vi "ClosedLoop+OpenWindLightOdor_v3.vi"() -> ()   [LabVIEW 2014]
uses:
  <vilib>/vision/Measure.llb/Straight Edge Options.ctl
  <vilib>/vision/Measure.llb/Straight Edge Process.ctl
  <vilib>/Platform/TimedLoop/XDataNode/timing_clust.ctl
  <vilib>/Platform/TimedLoop/XDataNode/nitl_modes.ctl
  <vilib>/Platform/TimedLoop/XDataNode/wakeup.ctl
  <vilib>/vision/Measure.llb/Edge Options.ctl
  <vilib>/vision/Measure.llb/Edge Polarity.ctl
  <vilib>/gmath/statdist.llb/Random Permutation.vi
  <vilib>/DAQmx/create/channels.llb/DAQmx Create Channel (DO-Digital Output).vi
  <vilib>/DAQmx/write.llb/DAQmx Write (Digital Bool 1Line 1Point).vi
  <vilib>/gmath/statdist.llb/Uniform (Discrete) Random.vi
  <vilib>/DAQmx/create/channels.llb/DAQmx Create Channel (AO-Voltage-Basic).vi
  <vilib>/Platform/TimedLoop/TimeConversion.llb/rt-rel-time-to-milliseconds.vi
  <vilib>/DAQmx/write.llb/DAQmx Write (Analog DBL 1Chan 1Samp).vi
  <vilib>/DAQmx/create/channels.llb/DAQmx Create Channel (DI-Digital Input).vi
  <vilib>/DAQmx/read.llb/DAQmx Read (Digital Bool 1Line 1Point).vi
  <vilib>/platform/TimedLoop/XDataNode/XDataNode.xnode
  <vilib>/vision/driver/NI_Vision_Acquisition_Software.lvlib
  <vilib>/Platform/TimedLoop/XDataNode/XDNodeRunTimeDep.lvlib
  <vilib>/vision/NI_Vision_Development_Module.lvlib
  <vilib>/gmath/NI_Gmath.lvlib
panel:
  out "Wind Intensity (V)":dbl=5.0
  out "Wind Trial":bool
  out "head ind":i32
  out "Slide 5":dbl(slide) scale=0.0..1.0
  out "Slide 4":dbl(slide) scale=0.0..1.0
  out "Slide 3":dbl(slide) scale=0.0..1.0
  out "Slide 2":dbl(slide) scale=0.0..1.0
  out "Light Trial":bool
  in  "Vary Stimulus Intensity":bool
  out "Cond. 4":i32
  out "Cond. 3":i32
  out "Cond. 2":i32
  out "Cond. 1":i32
  out "Light Intensity (V)":dbl=5.0
  in  "Rand light":bool
  in  "Use light?":bool
  in  "Reversed Tether?":bool=TRUE
  in  "R options":T1={"Number of Lines"=1, "Type"=enum."Best Edge Projection", "Min. Score"=10.0, "Max. Score"=1000.0, "Orientation"=-135.0, "Angle Range"=45.0, "Angle Tolerance"=1.0, "Step Size"=3, "Min. SNR (db)"=0.0, "Min. Points (%)"=25.0, "Hough Iterations"=3} {"Min. Points (%)" min=0.0 max=100.0; "Min. SNR (db)" min=0.0; "Max. Score" min=0.0 max=1024.0; "Min. Score" min=0.0 max=1024.0 step=1.0}
  in  "L options":T1={"Number of Lines"=1, "Type"=enum."Best Edge Projection", "Min. Score"=10.0, "Max. Score"=1000.0, "Orientation"=135.0, "Angle Range"=45.0, "Angle Tolerance"=1.0, "Step Size"=3, "Min. SNR (db)"=0.0, "Min. Points (%)"=25.0, "Hough Iterations"=3} {"Min. Points (%)" min=0.0 max=100.0; "Min. SNR (db)" min=0.0; "Max. Score" min=0.0 max=1024.0; "Min. Score" min=0.0 max=1024.0 step=1.0}
  in  "Rand wind":bool
  in  "Use wind?":bool=TRUE
  in  "Use odor?":bool
  in  "Pre-Spec. H(0)":bool=TRUE
  out "X (steps/sample)":dbl(graph)
  out "Slide":dbl(slide) scale=0.0..1.0
  out "Motor Error":bool
  in  "Max steps/sample":dbl=6.0
  in  "Step Rate (Hz)":dbl=500.0
  out "Heading (deg)":dbl(graph)
  out "H":dbl format="%.4f"
  out "X (steps/sample)":dbl
  in  "Geneotype":string="w1118"
  out "Odor On":bool
  in  "Starvation Time (hrs)":string="1"
  in  "Age (DSE)":string="4"
  out "Trial End":bool
  in  "Trial Duration (s)":dbl=60.0
  out "Odor Duration (s)":dbl=10.0
  in  "Odor Onset Time (s)":dbl=90.0
  out "Trial":i32 format="%#.3f"
  in  "Number of Trials":i32=20
  in  "Experiment name":string="E1"
  in  "Fly ID":string
  in  "L-R WBA Offset (deg)":dbl format="%#_13g"
  in  "deltaWBA Scale Factor (k, unitless)":dbl=0.04 format="%.4f"
  out "L-R WBA":dbl
  out "deltaWBA":dbl format="%.4f"
  out "Scaled deltaWBA (deg)":dbl(graph)
  out "R WBA":dbl
  out "L WBA":dbl
  out "Image":T3(plugin-control)
  in  "Image Threshold":cluster{"Lower value":sgl, "Upper value":sgl}={"Lower value"=110.0, "Upper value"=255.0} {"Upper value" format="%.2f"; "Lower value" format="%.2f"}
  in  "Data Rate (Hz)":dbl=50.0
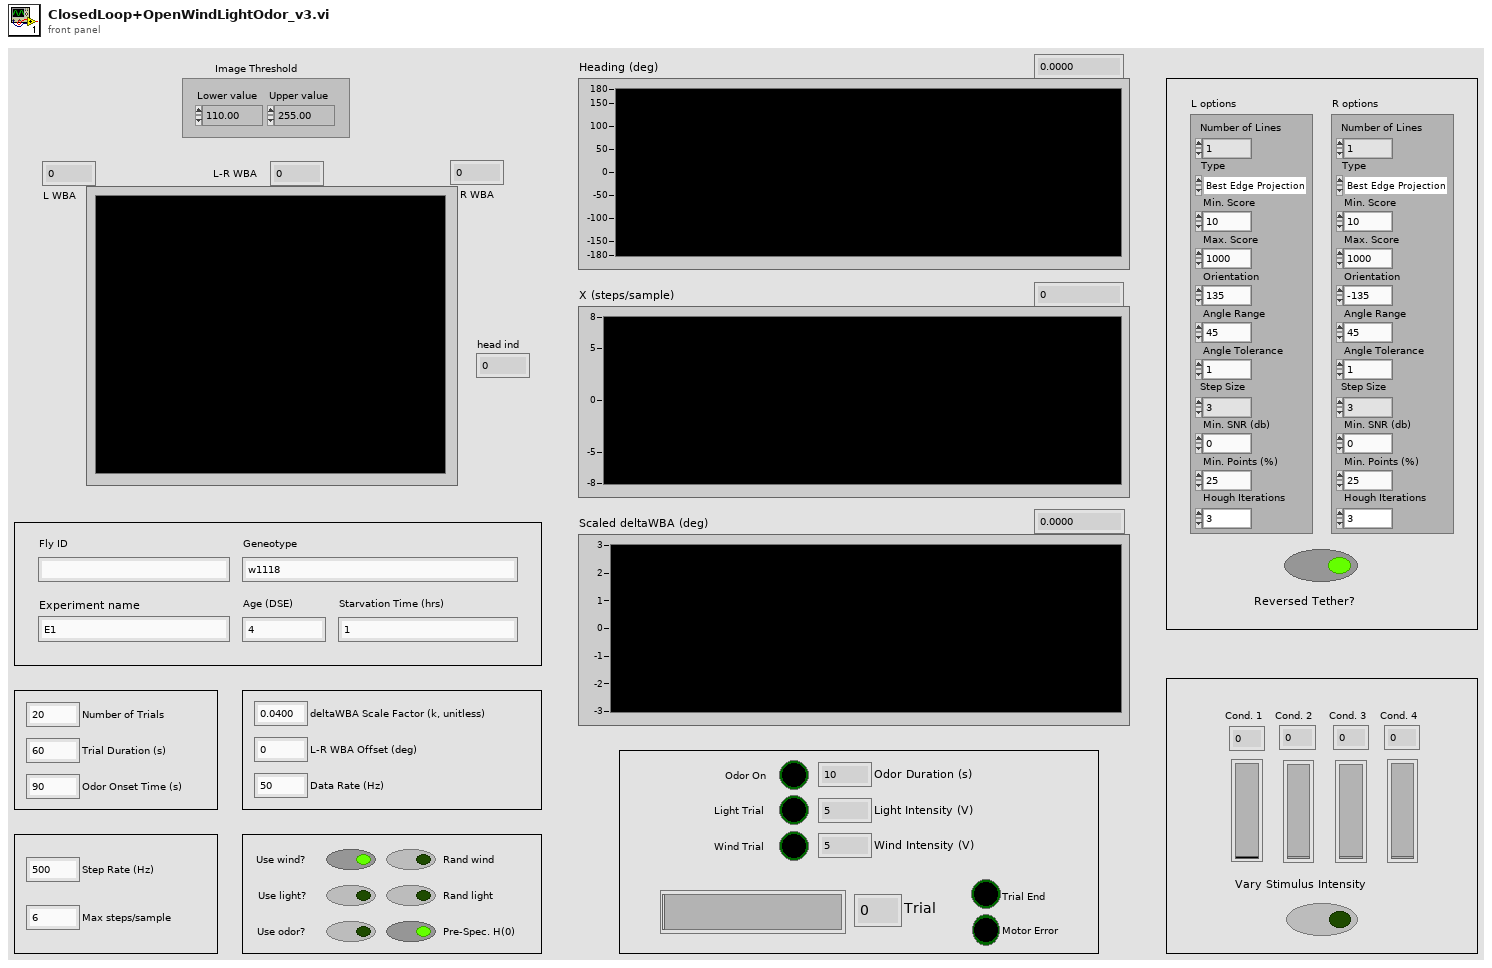
[diagram p1: front panel]
types:
  T1 = typedef "Straight Edge Options.ctl" = cluster{"Number of Lines":i32, "Type":T2, "Min. Score":dbl, "Max. Score":dbl, "Orientation":dbl, "Angle Range":dbl, "Angle Tolerance":dbl, "Step Size":u32, "Min. SNR (db)":dbl, "Min. Points (%)":dbl, "Hough Iterations":i32}
  T2 = typedef "Straight Edge Process.ctl" = enum32{"First Edge Rake", "Best Edge Rake", "Hough Edge Rake", "First Edge Projection", "Best Edge Projection"}
  T3 = typedef "IMAQ Image.ctl" = refnum<image>
  T4 = enum16{"open", "replace", "create", "open or create", "replace or create", "replace or create with confirmation"}
  T5 = typedef "IMAQdx.ctl" = refnum<k21>
  T6 = typedef "IMAQ Rectangle" = cluster{"Left":i32, "Top":i32, "Right":i32, "Bottom":i32, "Rotation":dbl}
  T7 = typedef "ROI Descriptor" = cluster{"Global Rectangle":i32[], "Contours":cluster{"ID":enum32{"External", "Internal"}, "Type":u32, "Coordinates":i32[]}[]}
  T8 = typedef "XDNodeRunTimeDep.lvlib/timing_clust.ctl" = cluster{"Expected End [f-1]":u64, "Actual End [f-1]":u64, "Finished Late? [f-1]":bool, "Expected End [i-1]":u64, "Actual End [i-1]":u64, "Finished Late? [i-1]":bool, "Expected Start [i]":u64, "Actual Start [i]":u64, "Expected Start [f]":u64, "Actual Start [f]":u64, "Source Name":string, "Structure Name":string, "Period":i64, "Deadline":i64, "Offset":i64, "Start":i64, "Priority":i32, "Timeout":i32, "Mode":T9, "Wakeup Reason":T10, "Error":errorcluster, "Source Type":string, "Secondary Source Type":string, "Global End Time":u64, "Global Start Time":u64, "Frame Duration":u64, "Iteration Duration":u64, "Assigned CPU":i32, "I/O Scan Engine Mode":u32}
  T9 = typedef "XDNodeRunTimeDep.lvlib/nitl_modes.ctl" = enum32{"No Change", "Process missed periods, maintain original phase", "Discard missed periods, maintain original phase", "Process missed periods, ignore original phase", "Discard missed periods, ignore original phase"}
  T10 = typedef "XDNodeRunTimeDep.lvlib/wakeup.ctl" = enum32{"Normal", "Aborted", "Asynchronous wakeup", "Timing source error", "Timed loop error", "Timeout"}
  T11 = typedef "Edge Options.ctl" = cluster{"Edge Polarity":T12, "Kernel Size":u32, "Width":u32, "Minimum Edge Strength":sgl, "Interpolation Type":enum32{"Zero Order", "Bilinear", "Quadratic", "Cubic", "Bilinear Fixed"}, "Data Processing Method":enum32{"Average", "Median"}}
  T12 = typedef "Edge Polarity.ctl" = u32
  T13 = cluster{"Search Direction":u32, "Edge Options":T11, "Show Search Area":bool, "Show Search Lines":bool, "Show Edges Found":bool, "Show Result":bool, "Search Area Color":u32, "Search Lines Color":u32, "Edge Locations Color":u32, "Result Color":u32, "Overlay Group Name":string}
  T14 = cluster{"Point1 (Pixels)":cluster{"X":sgl, "Y":sgl}, "Point2 (Pixels)":cluster{"X":sgl, "Y":sgl}, "Point1 (Real-World)":cluster{"X":sgl, "Y":sgl}, "Point2 (Real-World)":cluster{"X":sgl, "Y":sgl}, "Angle (Pixel)":dbl, "Angle (Real-World)":dbl, "Score":dbl, "Straightness":dbl, "Average SNR (db)":dbl, "Calibration Valid":bool}[]
  T15 = cluster{"Straight Edges[0]":cluster{"Point1 (Pixels)":cluster{"X":sgl, "Y":sgl}, "Point2 (Pixels)":cluster{"X":sgl, "Y":sgl}, "Point1 (Real-World)":cluster{"X":sgl, "Y":sgl}, "Point2 (Real-World)":cluster{"X":sgl, "Y":sgl}, "Angle (Pixel)":dbl, "Angle (Real-World)":dbl, "Score":dbl, "Straightness":dbl, "Average SNR (db)":dbl, "Calibration Valid":bool}, "Straight Edges[1]":cluster{"Point1 (Pixels)":cluster{"X":sgl, "Y":sgl}, "Point2 (Pixels)":cluster{"X":sgl, "Y":sgl}, "Point1 (Real-World)":cluster{"X":sgl, "Y":sgl}, "Point2 (Real-World)":cluster{"X":sgl, "Y":sgl}, "Angle (Pixel)":dbl, "Angle (Real-World)":dbl, "Score":dbl, "Straightness":dbl, "Average SNR (db)":dbl, "Calibration Valid":bool}, "Straight Edges[2]":cluster{"Point1 (Pixels)":cluster{"X":sgl, "Y":sgl}, "Point2 (Pixels)":cluster{"X":sgl, "Y":sgl}, "Point1 (Real-World)":cluster{"X":sgl, "Y":sgl}, "Point2 (Real-World)":cluster{"X":sgl, "Y":sgl}, "Angle (Pixel)":dbl, "Angle (Real-World)":dbl, "Score":dbl, "Straightness":dbl, "Average SNR (db)":dbl, "Calibration Valid":bool}, "Straight Edges[3]":cluster{"Point1 (Pixels)":cluster{"X":sgl, "Y":sgl}, "Point2 (Pixels)":cluster{"X":sgl, "Y":sgl}, "Point1 (Real-World)":cluster{"X":sgl, "Y":sgl}, "Point2 (Real-World)":cluster{"X":sgl, "Y":sgl}, "Angle (Pixel)":dbl, "Angle (Real-World)":dbl, "Score":dbl, "Straightness":dbl, "Average SNR (db)":dbl, "Calibration Valid":bool}, "Straight Edges[4]":cluster{"Point1 (Pixels)":cluster{"X":sgl, "Y":sgl}, "Point2 (Pixels)":cluster{"X":sgl, "Y":sgl}, "Point1 (Real-World)":cluster{"X":sgl, "Y":sgl}, "Point2 (Real-World)":cluster{"X":sgl, "Y":sgl}, "Angle (Pixel)":dbl, "Angle (Real-World)":dbl, "Score":dbl, "Straightness":dbl, "Average SNR (db)":dbl, "Calibration Valid":bool}, "Straight Edges[5]":cluster{"Point1 (Pixels)":cluster{"X":sgl, "Y":sgl}, "Point2 (Pixels)":cluster{"X":sgl, "Y":sgl}, "Point1 (Real-World)":cluster{"X":sgl, "Y":sgl}, "Point2 (Real-World)":cluster{"X":sgl, "Y":sgl}, "Angle (Pixel)":dbl, "Angle (Real-World)":dbl, "Score":dbl, "Straightness":dbl, "Average SNR (db)":dbl, "Calibration Valid":bool}, "Straight Edges[6]":cluster{"Point1 (Pixels)":cluster{"X":sgl, "Y":sgl}, "Point2 (Pixels)":cluster{"X":sgl, "Y":sgl}, "Point1 (Real-World)":cluster{"X":sgl, "Y":sgl}, "Point2 (Real-World)":cluster{"X":sgl, "Y":sgl}, "Angle (Pixel)":dbl, "Angle (Real-World)":dbl, "Score":dbl, "Straightness":dbl, "Average SNR (db)":dbl, "Calibration Valid":bool}, "Straight Edges[7]":cluster{"Point1 (Pixels)":cluster{"X":sgl, "Y":sgl}, "Point2 (Pixels)":cluster{"X":sgl, "Y":sgl}, "Point1 (Real-World)":cluster{"X":sgl, "Y":sgl}, "Point2 (Real-World)":cluster{"X":sgl, "Y":sgl}, "Angle (Pixel)":dbl, "Angle (Real-World)":dbl, "Score":dbl, "Straightness":dbl, "Average SNR (db)":dbl, "Calibration Valid":bool}, "Straight Edges[8]":cluster{"Point1 (Pixels)":cluster{"X":sgl, "Y":sgl}, "Point2 (Pixels)":cluster{"X":sgl, "Y":sgl}, "Point1 (Real-World)":cluster{"X":sgl, "Y":sgl}, "Point2 (Real-World)":cluster{"X":sgl, "Y":sgl}, "Angle (Pixel)":dbl, "Angle (Real-World)":dbl, "Score":dbl, "Straightness":dbl, "Average SNR (db)":dbl, "Calibration Valid":bool}}
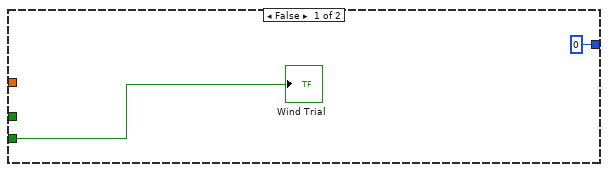
[diagram p2: hidden frame]
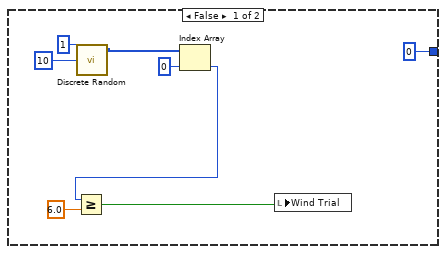
[diagram p3: hidden frame]
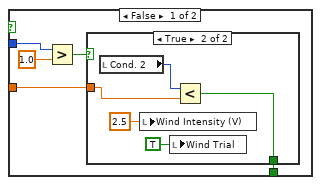
[diagram p4: hidden frame]
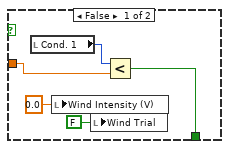
[diagram p5: hidden frame]
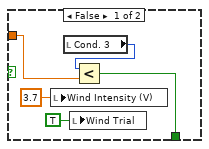
[diagram p6: hidden frame]
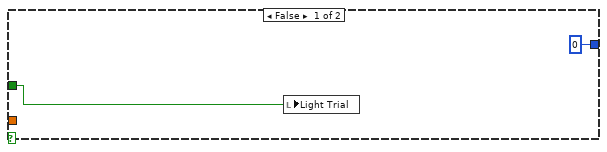
[diagram p7: hidden frame]
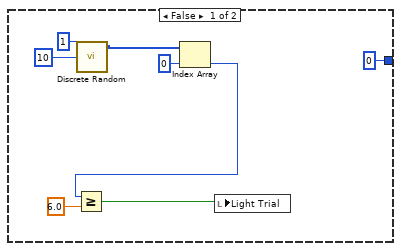
[diagram p8: hidden frame]
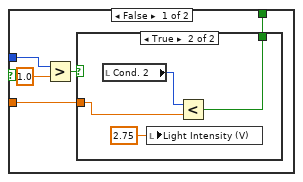
[diagram p9: hidden frame]
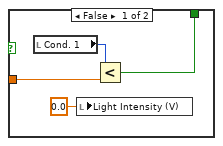
[diagram p10: hidden frame]
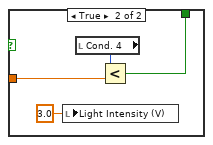
[diagram p11: hidden frame]
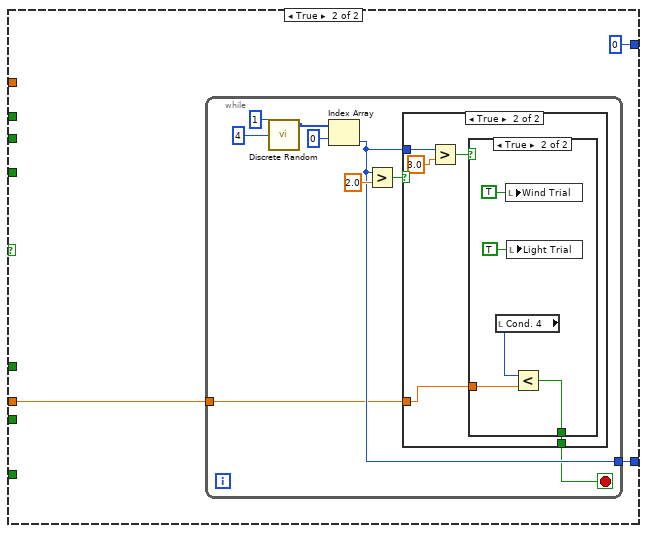
[diagram p12: hidden frame]
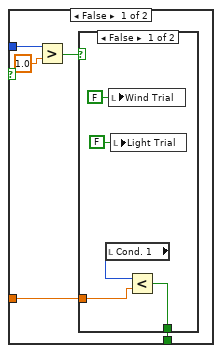
[diagram p13: hidden frame]
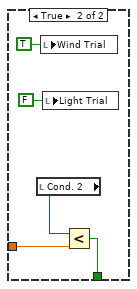
[diagram p14: hidden frame]
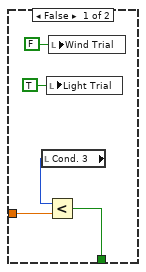
[diagram p15: hidden frame]
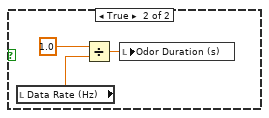
[diagram p17: hidden frame]
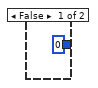
[diagram p19: hidden frame]
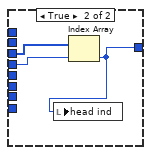
[diagram p20: hidden frame]
diagram:
  w123 = "."
  w125 = "."
  n1 = Boolean To (0,1)(Boolean="Use odor?") -> (0, 1=w86:i16)
  n2 = Boolean To (0,1)(Boolean="Use wind?") -> (0, 1=w75:i16)
  n3 = Boolean To (0,1)(Boolean="Vary Stimulus Intensity") -> (0, 1=w33:i16)
  n4 = Boolean To (0,1)(Boolean="Rand wind") -> (0, 1=w71:i16)
  n5 = Boolean To (0,1)(Boolean="Use light?") -> (0, 1=w50:i16)
  n6 = Boolean To (0,1)(Boolean="Rand light") -> (0, 1=w46:i16)
  n7 = local read "deltaWBA Scale Factor (k, unitless)"() -> (w100:dbl)
  n8 = local read "Data Rate (Hz)"() -> (w101:dbl)
  n9 = local read "Odor Onset Time (s)"() -> (w106:dbl)
  n10 = local read "Trial Duration (s)"() -> (w109:dbl)
  n11 = local read "Number of Trials"() -> (w111:i32)
  n12 = To Double Precision Float(number=w86) -> (double precision float=w85:dbl)
  n13 = To Double Precision Float(number=w75) -> (double precision float=w74:dbl)
  n14 = To Double Precision Float(number=w33) -> (double precision float=w31:dbl)
  n15 = To Double Precision Float(number=w71) -> (double precision float=w69:dbl)
  n16 = local read "Max steps/sample"() -> (w98:dbl)
  n17 = To Double Precision Float(number=w50) -> (double precision float=w48:dbl)
  n18 = To Double Precision Float(number=w46) -> (double precision float=w44:dbl)
  n19 = local read "Step Rate (Hz)"() -> (w99:dbl)
  n20 = local read "Reversed Tether?"() -> (w54:bool)
  n21 = Boolean To (0,1)(Boolean=w54) -> (0, 1=w55:i16)
  n22 = To Double Precision Float(number=w55) -> (double precision float=w53:dbl)
  n23 = Number To Fractional String(number=w111, precision (6)=i16 0) -> (F-format string=w92:string)  [unwired: 2 in]
  n24 = Number To Fractional String(number=w109, precision (6)=i16 0) -> (F-format string=w91:string)  [unwired: 2 in]
  n25 = Number To Fractional String(number=w106, precision (6)=i16 0) -> (F-format string=w90:string)  [unwired: 2 in]
  n26 = Number To Fractional String(number=w85, precision (6)=i16 0) -> (F-format string=w89:string)  [unwired: 2 in]
  n27 = Number To Fractional String(number=w74, precision (6)=i16 0) -> (F-format string=w73:string)  [unwired: 2 in]
  n28 = Number To Fractional String(number=w101, precision (6)=i16 0) -> (F-format string=w67:string)  [unwired: 2 in]
  n29 = Number To Fractional String(number=w99, precision (6)=i16 0) -> (F-format string=w66:string)  [unwired: 2 in]
  n30 = Number To Fractional String(number=w98, precision (6)=i16 0) -> (F-format string=w65:string)  [unwired: 2 in]
  n31 = Number To Fractional String(number=w100, precision (6)=i16 3) -> (F-format string=w64:string)  [unwired: 2 in]
  n32 = Number To Fractional String(number=w31, precision (6)=i16 0) -> (F-format string=w30:string)  [unwired: 2 in]
  n33 = Number To Fractional String(number=w69, precision (6)=i16 0) -> (F-format string=w68:string)  [unwired: 2 in]
  n34 = Number To Fractional String(number=w53, precision (6)=i16 0) -> (F-format string=w52:string)  [unwired: 2 in]
  n35 = Number To Fractional String(number=w48, precision (6)=i16 0) -> (F-format string=w36:string)  [unwired: 2 in]
  n36 = Number To Fractional String(number=w44, precision (6)=i16 0) -> (F-format string=w35:string)  [unwired: 2 in]
  n37 = Get Date/Time In Seconds() -> (seconds since 1Jan1904=w131:timestamp)
  n38 = Get Date/Time In Seconds() -> (seconds since 1Jan1904=w127:timestamp)
  n39 = Get Date/Time In Seconds() -> (seconds since 1Jan1904=w129:timestamp)
  n40 = call <vilib>:"Space Constant.vi"() -> ("String"=w133:string)
  n41 = Format Date/Time String(time format string (%c)="%d", seconds (now)=w131) -> (date/time string=w122:string)  [unwired: 1 in]
  n42 = Format Date/Time String(time format string (%c)="%m", seconds (now)=w129) -> (date/time string=w124:string)  [unwired: 1 in]
  n43 = Format Date/Time String(time format string (%c)="%Y", seconds (now)=w127) -> (date/time string=w126:string)  [unwired: 1 in]
  n44 = Concatenate Strings(w126, w125, w124, w123, w122) -> (w97:string)
  n45 = Concatenate Strings(w126, w125, w124, w123, w122, w133, "fly_", "Fly ID", "\\") -> (w137:string)
  n46 = String To Path(string=w137) -> (path=w136:path)
  n47 = Build Path(base path=path "E:/TAC DATA ARCHIVE/NewRig/labview/ClosedLoop+OpenWindLightOdor", name or relative path=w136) -> (appended path=w141:path)
  n48 = call <vilib>:"IMAQdx Open Camera.vi"("Session In"=refnum<k21> "cam8" ("Camera Name")) -> ("Session Out"=w163:T5)  [unwired: 2 in, 8 out]
  n49 = call <vilib>:"Check if File or Folder Exists.vi"("path"=w141) -> ("file or folder exists?"=w139:bool, "dup path"=w140:path)  [unwired: 8 in, 1 out]
  n50 = call <vilib>:"IMAQdx Configure Grab.vi"("Session In"=w163) -> ("Session Out"=w161:T5)  [unwired: 1 in, 9 out]
  n51 = case shown="False" w139 {
    tunnel: w140 -> [w165 w166]
    tunnel: [w164 w166] -> w145
    frame False {
      n52 = Create Folder(path (use dialog)=w165) -> (created path=w164:path)  [unwired: 2 in, 2 out]
    }
    frame True {
    }
  }
  n53 = call "IMAQ Create"("Image Name"="ROIR") -> ("New Image"=w160:T3)  [unwired: 3 in, 2 out]
  n54 = Concatenate Strings("Experiment name", "\\") -> (w113:string)
  n55 = call <vilib>:"IMAQdx Grab.vi"("Image In"=w160, "Session In"=w161) -> ("Image Out"=w159:T3, "Session Out"=w150:T5)  [unwired: 2 in, 6 out]
  n56 = String To Path(string=w113) -> (path=w142:path)
  n57 = call "IMAQ Select Rectangle"("Prompt"="Select RIGHT ROI for wing angle detection", "Image In"=w159) -> ("Rectangle"=w151:T6)  [unwired: 6 in, 3 out]
  n58 = Build Path(base path=w145, name or relative path=w142) -> (appended path=w146:path)
  n59 = call "IMAQ Convert Rectangle to ROI"("Rectangle"=w151) -> ("ROI Descriptor"=w149:T7)  [unwired: 8 in, 1 out]
  n60 = call <vilib>:"Check if File or Folder Exists.vi"("path"=w146) -> ("file or folder exists?"=w143:bool, "dup path"=w144:path)  [unwired: 8 in, 1 out]
  n61 = call "IMAQ Create"("Image Name"="ROIL") -> ("New Image"=w155:T3)  [unwired: 3 in, 2 out]
  n62 = case shown="False" w143 {
    tunnel: w144 -> [w168 w169]
    tunnel: [w167 w169] -> w1
    frame False {
      n63 = Create Folder(path (use dialog)=w168) -> (created path=w167:path)  [unwired: 2 in, 2 out]
    }
    frame True {
    }
  }
  n64 = call <vilib>:"IMAQdx Grab.vi"("Image In"=w155, "Session In"=w150) -> ("Image Out"=w154:T3, "Session Out"=w148:T5)  [unwired: 2 in, 6 out]
  n65 = String To Path(string="experiment_information") -> (path=w121:path)
  n66 = call "IMAQ Select Rectangle"("Prompt"="Select LEFT ROI for wing angle detection", "Image In"=w154) -> ("Rectangle"=w156:T6)  [unwired: 6 in, 3 out]
  n67 = Build Path(base path=w1, name or relative path=w121) -> (appended path=w118:path)
  n68 = String To Path(string="odor_durations") -> (path=w84:path)
  n69 = String To Path(string="light_intensities") -> (path=w43:path)
  n70 = String To Path(string="wind_boolean") -> (path=w63:path)
  n71 = String To Path(string="wind_intensities") -> (path=w10:path)
  n72 = call "IMAQ Convert Rectangle to ROI"("Rectangle"=w156) -> ("ROI Descriptor"=w147:T7)  [unwired: 8 in, 1 out]
  n73 = Build Path(base path=w1, name or relative path=w84) -> (appended path=w81:path)
  n74 = Build Path(base path=w1, name or relative path=w43) -> (appended path=w40:path)
  n75 = Build Path(base path=w1, name or relative path=w63) -> (appended path=w60:path)
  n76 = Build Path(base path=w1, name or relative path=w10) -> (appended path=w7:path)
  n77 = Open/Create/Replace File(file path (use dialog)=w118, operation (0:open)=T4."create", access (0:read/write)=enum16{"read/write", "read-only", "write-only"}."write-only") -> (refnum out=w116:refnum<file>)  [unwired: 3 in, 2 out]
  n78 = Open/Create/Replace File(file path (use dialog)=w81, operation (0:open)=T4."create", access (0:read/write)=enum16{"read/write", "read-only", "write-only"}."write-only") -> (refnum out=w79:refnum<file>)  [unwired: 3 in, 2 out]
  n79 = Open/Create/Replace File(file path (use dialog)=w40, operation (0:open)=T4."create", access (0:read/write)=enum16{"read/write", "read-only", "write-only"}."write-only") -> (refnum out=w38:refnum<file>)  [unwired: 3 in, 2 out]
  n80 = Open/Create/Replace File(file path (use dialog)=w60, operation (0:open)=T4."create", access (0:read/write)=enum16{"read/write", "read-only", "write-only"}."write-only") -> (refnum out=w58:refnum<file>)  [unwired: 3 in, 2 out]
  n81 = Open/Create/Replace File(file path (use dialog)=w7, operation (0:open)=T4."create", access (0:read/write)=enum16{"read/write", "read-only", "write-only"}."write-only") -> (refnum out=w5:refnum<file>)  [unwired: 3 in, 2 out]
  n82 = Build Array(w97, "Fly ID", "Experiment name", "Age (DSE)", "Starvation Time (hrs)", w92, w91, w90, w89, w73, w68, w67, w66, w65, w64, w52, w36, w35, w30, "Geneotype") -> (w88:string[])
  n83 = Write to Text File(file (use dialog)=w116, text=w88) -> (refnum out=w115:refnum<file>)  [unwired: 2 in, 2 out]
  n84 = Close File(refnum=w115) -> ()  [unwired: 1 in, 2 out]
  n85 = flat-sequence {
    tunnel: w1 -> [w175]
    tunnel: w147 -> [w176]
    tunnel: w148 -> [w177]
    tunnel: w149 -> [w178]
    tunnel: [w178] -> w28
    tunnel: [w177] -> w26
    tunnel: [w176] -> w24
    tunnel: [w175] -> w22
    tunnel: [w173] -> w20
    tunnel: w79 -> [w173]
    tunnel: [w172] -> w18
    tunnel: w58 -> [w172]
    tunnel: w38 -> [w171]
    tunnel: [w171] -> w16
    tunnel: w5 -> [w170]
    tunnel: [w170] -> w4
    tunnel: w28 -> [w193]
    tunnel: [w193] -> w27
    tunnel: w26 -> [w192]
    tunnel: [w192] -> w25
    tunnel: w24 -> [w191]
    tunnel: [w191] -> w23
    tunnel: w22 -> [w190]
    tunnel: [w190] -> w21
    tunnel: w20 -> [w189]
    tunnel: [w189] -> w19
    tunnel: w18 -> [w188]
    tunnel: [w188] -> w17
    tunnel: w16 -> [w187]
    tunnel: [w187] -> w15
    tunnel: [w186] -> w14
    tunnel: [w185] -> w13
    tunnel: [w184] -> w12
    tunnel: [w183] -> w11
    tunnel: w4 -> [w179]
    tunnel: [w179] -> w3
    tunnel: w27 -> [w214]
    tunnel: w25 -> [w213]
    tunnel: w23 -> [w212]
    tunnel: w21 -> [w211]
    tunnel: w19 -> [w209]
    tunnel: [w208] -> w78
    tunnel: w17 -> [w207]
    tunnel: [w206] -> w57
    tunnel: w15 -> [w205]
    tunnel: [w204] -> w37
    tunnel: w14 -> [w199]
    tunnel: w13 -> [w198]
    tunnel: w12 -> [w197]
    tunnel: w11 -> [w196]
    tunnel: w3 -> [w195]
    tunnel: [w194] -> w2
    tunnel: w78 -> [w1391]
    tunnel: w57 -> [w1390]
    tunnel: w37 -> [w1389]
    tunnel: w2 -> [w1388]
    frame #0 {
      n86 = One Button Dialog(message="Ensure the stage is at 0 degrees.") -> ()  [unwired: 1 in, 1 out]
    }
    frame #1 {
      n87 = local read "Number of Trials"() -> (w182:i32)
      n88 = Divide(x=w182, y=4) -> (x/y=w180:dbl)
      n89 = call-poly <vilib>:"Discrete Random.vi"("N"=w180) -> ("random permutation"=w186:i32[])  [unwired: 9 in, 1 out]
      n90 = call-poly <vilib>:"Discrete Random.vi"("N"=w180) -> ("random permutation"=w185:i32[])  [unwired: 9 in, 1 out]
      n91 = call-poly <vilib>:"Discrete Random.vi"("N"=w180) -> ("random permutation"=w183:i32[])  [unwired: 9 in, 1 out]
      n92 = call-poly <vilib>:"Discrete Random.vi"("N"=w180) -> ("random permutation"=w184:i32[])  [unwired: 9 in, 1 out]
    }
    frame #2 {
      n93 = for {
        N: "Number of Trials" -> [_]
        tunnel: w214 -> [w312]
        tunnel: w213 -> [w311]
        tunnel: w212 -> [w310]
        tunnel: w211 -> [w309]
        shift-right: [w289] -> w208
        shift-left: w209 -> [w293]
        shift-right: [w283] -> w206
        shift-left: w207 -> [w287]
        shift-right: [w278] -> w204
        shift-left: w205 -> [w282]
        shift-right: [w270] -> _
        shift-left: 0 ("y") -> [w264]
        shift-right: [w269] -> _
        shift-left: 0 ("y") -> [w262]
        shift-right: [w268] -> _
        shift-left: 0 ("y") -> [w260]
        shift-right: [w267] -> _
        shift-left: 0 ("y") -> [w258]
        tunnel: w199 -> [w255]
        tunnel: w198 -> [w254]
        tunnel: w197 -> [w253]
        tunnel: w196 -> [w252]
        shift-right: [w216] -> w194
        shift-left: w195 -> [w222]
        i -> [w306]
        n94 = local read "Number of Trials"() -> (w266:i32)
        n95 = local read "Number of Trials"() -> (w297:i32)
        n96 = Divide(x=w266, y=4) -> (x/y=w257:dbl)
        n97 = Divide(x=w264, y=w257) -> (x/y=→"Slide 2":dbl)
        n98 = Divide(x=w260, y=w257) -> (x/y=→"Slide 4":dbl)
        n99 = Divide(x=w262, y=w257) -> (x/y=→"Slide 3":dbl)
        n100 = Divide(x=w258, y=w257) -> (x/y=→"Slide 5":dbl)
        n101 = flat-sequence {
          tunnel: w296 -> [w349]
          tunnel: w309 -> [w350]
          tunnel: w310 -> [w351]
          tunnel: w311 -> [w352]
          tunnel: w312 -> [w353]
          tunnel: [w353] -> w251
          tunnel: [w352] -> w249
          tunnel: [w351] -> w247
          tunnel: [w350] -> w245
          tunnel: [w349] -> w243
          tunnel: [w340] -> w241
          tunnel: w293 -> [w340]
          tunnel: w287 -> [w337]
          tunnel: [w337] -> w239
          tunnel: [w334] -> w237
          tunnel: w282 -> [w334]
          tunnel: [w330] -> w235
          tunnel: w260 -> [w324]
          tunnel: w258 -> [w322]
          tunnel: w262 -> [w326]
          tunnel: w264 -> [w328]
          tunnel: w257 -> [w321]
          tunnel: w255 -> [w329]
          tunnel: w254 -> [w327]
          tunnel: w253 -> [w325]
          tunnel: w252 -> [w323]
          tunnel: [w329] -> w232
          tunnel: [w328] -> w231
          tunnel: [w327] -> w230
          tunnel: [w326] -> w229
          tunnel: [w325] -> w228
          tunnel: [w324] -> w227
          tunnel: [w323] -> w226
          tunnel: [w322] -> w225
          tunnel: [w319] -> w223
          tunnel: w222 -> [w318]
          tunnel: [w318] -> w221
          tunnel: w251 -> [w547]
          tunnel: [w547] -> w250
          tunnel: w249 -> [w546]
          tunnel: [w546] -> w248
          tunnel: w247 -> [w545]
          tunnel: [w545] -> w246
          tunnel: w245 -> [w544]
          tunnel: [w544] -> w244
          tunnel: w243 -> [w543]
          tunnel: [w543] -> w242
          tunnel: w241 -> [w542]
          tunnel: [w542] -> w240
          tunnel: w239 -> [w541]
          tunnel: [w541] -> w238
          tunnel: w237 -> [w540]
          tunnel: [w540] -> w236
          tunnel: w235 -> [w527]
          tunnel: [w525] -> w234
          tunnel: [w539] -> w233
          tunnel: w232 -> [w535]
          tunnel: w231 -> [w537]
          tunnel: w230 -> [w534]
          tunnel: w229 -> [w536]
          tunnel: w228 -> [w533]
          tunnel: w227 -> [w532]
          tunnel: w226 -> [w531]
          tunnel: w225 -> [w530]
          tunnel: [w529] -> w224
          tunnel: w223 -> [w526]
          tunnel: w221 -> [w524]
          tunnel: [w524] -> w220
          tunnel: [w522] -> w215
          tunnel: [w680] -> w317
          tunnel: [w679] -> w316
          tunnel: [w678] -> w315
          tunnel: [w647] -> w314
          tunnel: w250 -> [w680]
          tunnel: w248 -> [w679]
          tunnel: w246 -> [w678]
          tunnel: w244 -> [w624]
          tunnel: w242 -> [w623]
          tunnel: [w646] -> w305
          tunnel: [w645] -> w302
          tunnel: [w622] -> w301
          tunnel: [w621] -> w300
          tunnel: [w619] -> w294
          tunnel: w240 -> [w618]
          tunnel: [w616] -> w292
          tunnel: w238 -> [w615]
          tunnel: [w613] -> w286
          tunnel: w236 -> [w612]
          tunnel: [w609] -> w281
          tunnel: w234 -> [w608]
          tunnel: [w608] -> w276
          tunnel: w233 -> [w607]
          tunnel: [w607] -> w273
          tunnel: w224 -> [w605]
          tunnel: w220 -> [w604]
          tunnel: [w601] -> w217
          tunnel: w215 -> [w599]
          tunnel: w317 -> [w959]
          tunnel: w316 -> [w958]
          tunnel: w315 -> [w957]
          tunnel: w314 -> [w956]
          tunnel: [w955] -> w313
          tunnel: [w952] -> w308
          tunnel: [w951] -> w307
          tunnel: w305 -> [w950]
          tunnel: [w949] -> w304
          tunnel: [w948] -> w303
          tunnel: w302 -> [w947]
          tunnel: w301 -> [w946]
          tunnel: w300 -> [w945]
          tunnel: [w944] -> w299
          tunnel: [w943] -> w298
          tunnel: w294 -> [w936]
          tunnel: w292 -> [w931]
          tunnel: [w931] -> w290
          tunnel: [w933] -> w288
          tunnel: w286 -> [w932]
          tunnel: [w932] -> w285
          tunnel: w281 -> [w928]
          tunnel: [w928] -> w279
          tunnel: [w927] -> w277
          tunnel: w276 -> [w926]
          tunnel: [w926] -> w274
          tunnel: w273 -> [w925]
          tunnel: [w925] -> w272
          tunnel: [w924] -> w218
          tunnel: w217 -> [w924]
          tunnel: w313 -> [w1202]
          tunnel: w308 -> [w1205]
          tunnel: w307 -> [w1204]
          tunnel: w304 -> [w1203]
          tunnel: w303 -> [w1201]
          tunnel: w299 -> [w1200]
          tunnel: w298 -> [w1199]
          tunnel: [w1196] -> w291
          tunnel: w290 -> [w1196]
          tunnel: w288 -> [w1194]
          tunnel: w285 -> [w1191]
          tunnel: [w1191] -> w284
          tunnel: [w1189] -> w280
          tunnel: w279 -> [w1189]
          tunnel: w277 -> [w1186]
          tunnel: [w1184] -> w275
          tunnel: w274 -> [w1184]
          tunnel: w272 -> [w1183]
          tunnel: [w1183] -> w271
          tunnel: [w1180] -> w219
          tunnel: w218 -> [w1180]
          tunnel: [w1318] -> w289
          tunnel: w291 -> [w1318]
          tunnel: w284 -> [w1317]
          tunnel: [w1317] -> w283
          tunnel: [w1316] -> w278
          tunnel: w280 -> [w1316]
          tunnel: w275 -> [w1309]
          tunnel: w271 -> [w1315]
          tunnel: [w1314] -> w270
          tunnel: [w1313] -> w269
          tunnel: [w1312] -> w268
          tunnel: [w1311] -> w267
          tunnel: [w1308] -> w216
          tunnel: w219 -> [w1308]
          frame #0 {
            n102 = local read "Rand wind"() -> (w339:bool)
            n103 = local read "Vary Stimulus Intensity"() -> (w320:bool)
            n104 = local read "Use light?"() -> (w335:bool)
            n105 = local read "Rand light"() -> (w336:bool)
            n106 = local read "Use wind?"() -> (w338:bool)
            n107 = And(x=w338, y=w339) -> (x .and. y?=w331:bool)
            n108 = And(x=w335, y=w336) -> (x .and. y?=w332:bool)
            n109 = And(x=w331, y=w332) -> (x .and. y?=w333:bool)
            n110 = case shown="False" w333 {
              tunnel: w331 -> [w358 _]
              tunnel: w338 -> [w357 _]
              tunnel: w332 -> [w363 _]
              tunnel: w335 -> [w362 _]
              tunnel: [w359 w471] -> w330
              tunnel: w321 -> [w360 w470]
              tunnel: w320 -> [w361 _]
              tunnel: w321 -> [w356 _]
              tunnel: w320 -> [w355 _]
              tunnel: [w354 0 ("Numeric")] -> w319
              frame False {
                n111 = case shown="True" w358 {
                  tunnel: w357 -> [w365 _]
                  tunnel: w356 -> [_ w368]
                  tunnel: w355 -> [_ w367]
                  tunnel: [0 ("Numeric") w366] -> w354
                  frame False {
                    "Wind Trial" <- w365
                  }
                  frame True {
                    n112 = case shown="True" w367 {
                      tunnel: w368 -> [_ w378]
                      tunnel: [0 ("Numeric") w377] -> w366
                      frame False {
                        n113 = call-poly <vilib>:"Discrete Random.vi"("n"=10, "samples"=1) -> ("uniform (discrete) random data"=w374:i32[])  [unwired: 8 in, 1 out]
                        n114 = Index Array(array=w374, index=0) -> (element=w371:i32)
                        n115 = Greater Or Equal?(x=w371, y=6.0) -> (x >= y?=w370:bool)
                        n116 = local write "Wind Trial"(w370) -> ()
                      }
                      frame True {
                        n117 = while {
                          tunnel: w378 -> [w384]
                          tunnel: [w380] -> w377
                          stop <- w381 stop-if-true
                          n118 = call-poly <vilib>:"Discrete Random.vi"("n"=4, "samples"=1) -> ("uniform (discrete) random data"=w385:i32[])  [unwired: 8 in, 1 out]
                          n119 = local write "Light Intensity (V)"(0.0 ("Light Intensity (V)")) -> ()
                          n120 = Index Array(array=w385, index=0) -> (element=w380:i32)
                          n121 = Greater?(x=w380, y=2.0) -> (0:w382:bool)
                          n122 = case shown="True" w382 {
                            tunnel: w384 -> [w390 w405]
                            tunnel: w380 -> [w392 w407]
                            tunnel: [w389 w404] -> w381
                            frame False {
                              n123 = Greater?(x=w392, y=1.0) -> (0:w391:bool)
                              n124 = case shown="True" w391 {
                                tunnel: w390 -> [w397 w402]
                                tunnel: [w396 w401] -> w389
                                frame False {
                                n125 = local read "Cond. 1"() -> (w398:i32)
                                n126 = local write "Wind Intensity (V)"(0.0 ("Wind Intensity (V)")) -> ()
                                n127 = local write "Wind Trial"(FALSE ("Wind Trial")) -> ()
                                n128 = Less?(x=w398, y=w397) -> (x < y?=w396:bool)
                                }
                                frame True {
                                n129 = local read "Cond. 2"() -> (w403:i32)
                                n130 = local write "Wind Intensity (V)"(2.5 ("Wind Intensity (V)")) -> ()
                                n131 = local write "Wind Trial"(TRUE ("Wind Trial")) -> ()
                                n132 = Less?(x=w403, y=w402) -> (x < y?=w401:bool)
                                }
                              }
                            }
                            frame True {
                              n133 = Greater?(x=w407, y=3.0) -> (0:w406:bool)
                              n134 = case shown="True" w406 {
                                tunnel: w405 -> [w412 w417]
                                tunnel: [w411 w416] -> w404
                                frame False {
                                n135 = local write "Wind Intensity (V)"(3.7 ("Wind Intensity (V)")) -> ()
                                n136 = local read "Cond. 3"() -> (w413:i32)
                                n137 = local write "Wind Trial"(TRUE ("Wind Trial")) -> ()
                                n138 = Less?(x=w413, y=w412) -> (x < y?=w411:bool)
                                }
                                frame True {
                                n139 = local read "Cond. 4"() -> (w418:i32)
                                n140 = local write "Wind Trial"(TRUE ("Wind Trial")) -> ()
                                n141 = Less?(x=w418, y=w417) -> (x < y?=w416:bool)
                                "Wind Intensity (V)" <- 5.0 ("Wind Intensity (V)")
                                }
                              }
                            }
                          }
                        }
                      }
                    }
                  }
                }
                n142 = case shown="True" w363 {
                  tunnel: w362 -> [w419 _]
                  tunnel: w361 -> [_ w423]
                  tunnel: w360 -> [_ w422]
                  tunnel: [0 ("Numeric") w421] -> w359
                  frame False {
                    n143 = local write "Light Trial"(w419) -> ()
                  }
                  frame True {
                    n144 = case shown="True" w423 {
                      tunnel: w422 -> [_ w433]
                      tunnel: [0 ("Numeric") w432] -> w421
                      frame False {
                        n145 = call-poly <vilib>:"Discrete Random.vi"("n"=10, "samples"=1) -> ("uniform (discrete) random data"=w429:i32[])  [unwired: 8 in, 1 out]
                        n146 = Index Array(array=w429, index=0) -> (element=w427:i32)
                        n147 = Greater Or Equal?(x=w427, y=6.0) -> (x >= y?=w424:bool)
                        n148 = local write "Light Trial"(w424) -> ()
                      }
                      frame True {
                        n149 = while {
                          tunnel: w433 -> [w435]
                          tunnel: [w436] -> w432
                          stop <- w434 stop-if-true
                          n150 = call-poly <vilib>:"Discrete Random.vi"("n"=4, "samples"=1) -> ("uniform (discrete) random data"=w439:i32[])  [unwired: 8 in, 1 out]
                          n151 = Index Array(array=w439, index=0) -> (element=w436:i32)
                          n152 = Greater?(x=w436, y=2.0) -> (0:w437:bool)
                          n153 = case shown="True" w437 {
                            tunnel: w436 -> [w446 w459]
                            tunnel: w435 -> [w444 w457]
                            tunnel: [w443 w456] -> w434
                            frame False {
                              n154 = Greater?(x=w446, y=1.0) -> (0:w445:bool)
                              n155 = case shown="True" w445 {
                                tunnel: w444 -> [w450 w454]
                                tunnel: [w449 w453] -> w443
                                frame False {
                                n156 = local read "Cond. 1"() -> (w451:i32)
                                n157 = local write "Light Intensity (V)"(0.0 ("Light Intensity (V)")) -> ()
                                n158 = Less?(x=w451, y=w450) -> (x < y?=w449:bool)
                                }
                                frame True {
                                n159 = local read "Cond. 2"() -> (w455:i32)
                                n160 = local write "Light Intensity (V)"(2.75 ("Light Intensity (V)")) -> ()
                                n161 = Less?(x=w455, y=w454) -> (x < y?=w453:bool)
                                }
                              }
                            }
                            frame True {
                              n162 = Greater?(x=w459, y=3.0) -> (0:w458:bool)
                              n163 = case shown="False" w458 {
                                tunnel: w457 -> [w463 w467]
                                tunnel: [w462 w466] -> w456
                                frame False {
                                n164 = local read "Cond. 3"() -> (w464:i32)
                                n165 = local write "Light Intensity (V)"(2.9 ("Light Intensity (V)")) -> ()
                                n166 = Less?(x=w464, y=w463) -> (x < y?=w462:bool)
                                }
                                frame True {
                                n167 = local write "Light Intensity (V)"(3.0 ("Light Intensity (V)")) -> ()
                                n168 = local read "Cond. 4"() -> (w468:i32)
                                n169 = Less?(x=w468, y=w467) -> (x < y?=w466:bool)
                                }
                              }
                            }
                          }
                        }
                      }
                    }
                  }
                }
              }
              frame True {
                n170 = while {
                  tunnel: [w474] -> w471
                  tunnel: w470 -> [w473]
                  stop <- w472 stop-if-true
                  n171 = call-poly <vilib>:"Discrete Random.vi"("n"=4, "samples"=1) -> ("uniform (discrete) random data"=w480:i32[])  [unwired: 8 in, 1 out]
                  n172 = Index Array(array=w480, index=0) -> (element=w474:i32)
                  n173 = Greater?(x=w474, y=2.0) -> (0:w476:bool)
                  n174 = case shown="True" w476 {
                    tunnel: w474 -> [w484 w499]
                    tunnel: w473 -> [w482 w497]
                    tunnel: [w481 w496] -> w472
                    frame False {
                      n175 = Greater?(x=w484, y=1.0) -> (0:w483:bool)
                      n176 = case shown="False" w483 {
                        tunnel: w482 -> [w489 w495]
                        tunnel: [w488 w493] -> w481
                        frame False {
                          n177 = local read "Cond. 1"() -> (w490:i32)
                          n178 = local write "Wind Trial"(FALSE ("Wind Trial")) -> ()
                          n179 = local write "Light Trial"(FALSE ("Light Trial")) -> ()
                          n180 = Less?(x=w490, y=w489) -> (x < y?=w488:bool)
                        }
                        frame True {
                          n181 = local read "Cond. 2"() -> (w494:i32)
                          n182 = local write "Wind Trial"(TRUE ("Wind Trial")) -> ()
                          n183 = local write "Light Trial"(FALSE ("Light Trial")) -> ()
                          n184 = Less?(x=w494, y=w495) -> (x < y?=w493:bool)
                        }
                      }
                    }
                    frame True {
                      n185 = Greater?(x=w499, y=3.0) -> (0:w498:bool)
                      n186 = case shown="True" w498 {
                        tunnel: w497 -> [w505 w510]
                        tunnel: [w503 w508] -> w496
                        frame False {
                          n187 = local read "Cond. 3"() -> (w504:i32)
                          n188 = local write "Light Trial"(TRUE ("Light Trial")) -> ()
                          n189 = Less?(x=w504, y=w505) -> (x < y?=w503:bool)
                          n190 = local write "Wind Trial"(FALSE ("Wind Trial")) -> ()
                        }
                        frame True {
                          n191 = local read "Cond. 4"() -> (w509:i32)
                          n192 = local write "Wind Trial"(TRUE ("Wind Trial")) -> ()
                          n193 = local write "Light Trial"(TRUE ("Light Trial")) -> ()
                          n194 = Less?(x=w509, y=w510) -> (x < y?=w508:bool)
                        }
                      }
                    }
                  }
                }
              }
            }
            n195 = local read "Use odor?"() -> (w341:bool)
            n196 = case shown="True" w341 {
              frame False {
              }
              frame True {
                n197 = call-poly <vilib>:"Discrete Random.vi"("n"=3, "samples"=1) -> ("uniform (discrete) random data"=w514:i32[])  [unwired: 8 in, 1 out]
                n198 = Index Array(array=w514, index=0) -> (element=w511:i32)
                n199 = Equal?(x=w511, y=1) -> (x = y?=w513:bool)
                n200 = case shown="False" w513 {
                  frame False {
                    n201 = local write "Odor Duration (s)"(10.0 ("Odor Duration (s)")) -> ()
                  }
                  frame True {
                    n202 = local read "Data Rate (Hz)"() -> (w520:dbl)
                    n203 = Divide(x=1.0, y=w520) -> (x/y=w521:dbl)
                    n204 = local write "Odor Duration (s)"(w521) -> ()
                  }
                }
              }
            }
            n205 = local write "Motor Error"(FALSE ("Trial End")) -> ()
            n206 = call-poly <vilib>:"DAQmx Create Virtual Channel.vi"("lines"=tag "Dev1/port0/line0") -> ("task out"=w347:refnum<k21>)  [unwired: 13 in, 1 out]
            n207 = local write "Trial End"(FALSE ("Trial End")) -> ()
            n208 = call <vilib>:"DAQmx Start Task.vi"("task/channels in"=w347) -> ("task out"=w346:refnum<k21>)  [unwired: 13 in, 1 out]
            n209 = call-poly <vilib>:"DAQmx Write.vi"("task/channels in"=w346, "data"=FALSE) -> ("task out"=w345:refnum<k21>)  [unwired: 11 in, 2 out]
            n210 = call <vilib>:"DAQmx Stop Task.vi"("task/channels in"=w345) -> ()  [unwired: 13 in, 2 out]
          }
          frame #1 {
            n211 = Greater Or Equal?(x=w527, y=w526) -> (x >= y?=w528:bool)
            n212 = case shown="False" w528 {
              tunnel: w526 -> [w548 _]
              tunnel: w527 -> [_ w549]
              tunnel: [w548 w549] -> w525
              frame False {
              }
              frame True {
              }
            }
            n213 = Greater Than 0?(x=w525) -> (x > 0?=w538:bool)
            n214 = case shown="True" w538 {
              tunnel: w537 -> [_ w558]
              tunnel: w536 -> [_ w556]
              tunnel: w535 -> [_ w559]
              tunnel: w534 -> [_ w557]
              tunnel: w533 -> [_ w555]
              tunnel: w532 -> [_ w554]
              tunnel: w531 -> [_ w553]
              tunnel: w530 -> [_ w552]
              tunnel: w525 -> [_ w560]
              tunnel: [0 ("random permutation") w551] -> w529
              frame False {
              }
              frame True {
                n215 = Greater?(x=w560, y=2.0) -> (0:w561:bool)
                n216 = case shown="False" w561 {
                  tunnel: w560 -> [w572 w590]
                  tunnel: w559 -> [w571 w589]
                  tunnel: w558 -> [w570 w588]
                  tunnel: w557 -> [w569 w587]
                  tunnel: w556 -> [w568 w586]
                  tunnel: w555 -> [w567 w585]
                  tunnel: w554 -> [w566 w584]
                  tunnel: w553 -> [w565 w583]
                  tunnel: w552 -> [w564 w582]
                  tunnel: [w563 w581] -> w551
                  frame False {
                    n217 = Greater?(x=w572, y=1.0) -> (0:w573:bool)
                    n218 = case shown="False" w573 {
                      tunnel: w571 -> [w577 _]
                      tunnel: w570 -> [w576 _]
                      tunnel: w569 -> [_ w580]
                      tunnel: w568 -> [_ w579]
                      tunnel: w567 -> [_ _]
                      tunnel: w566 -> [_ _]
                      tunnel: w565 -> [_ _]
                      tunnel: w564 -> [_ _]
                      tunnel: [w575 w578] -> w563
                      frame False {
                        n219 = Index Array(array=w577, index=w576) -> (element=w575:i32)
                        "head ind" <- w575
                      }
                      frame True {
                        n220 = Index Array(array=w580, index=w579) -> (element=w578:i32)
                        n221 = local write "head ind"(w578) -> ()
                      }
                    }
                  }
                  frame True {
                    n222 = Greater?(x=w590, y=3.0) -> (0:w591:bool)
                    n223 = case shown="False" w591 {
                      tunnel: w589 -> [_ _]
                      tunnel: w588 -> [_ _]
                      tunnel: w587 -> [_ _]
                      tunnel: w586 -> [_ _]
                      tunnel: w585 -> [w595 _]
                      tunnel: w584 -> [w594 _]
                      tunnel: w583 -> [_ w598]
                      tunnel: w582 -> [_ w597]
                      tunnel: [w593 w596] -> w581
                      frame False {
                        n224 = Index Array(array=w595, index=w594) -> (element=w593:i32)
                        n225 = local write "head ind"(w593) -> ()
                      }
                      frame True {
                        n226 = Index Array(array=w598, index=w597) -> (element=w596:i32)
                        n227 = local write "head ind"(w596) -> ()
                      }
                    }
                  }
                }
              }
            }
            n228 = call-poly <vilib>:"DAQmx Create Virtual Channel.vi"("physical channels"=tag "Dev1/ao1") -> ("task out"=w522:refnum<k21>)  [unwired: 13 in, 1 out]
            n229 = Bundle("y"=w537, "y"=w536, "y"=w532, "y"=w530) -> (w539:cluster{"y":i32, "y":i32, "y":i32, "y":i32})  [unwired: 1 in]
          }
          frame #2 {
            n230 = local read "Vary Stimulus Intensity"() -> (w606:bool)
            n231 = local read "Odor Duration (s)"() -> (w617:dbl)
            n232 = case shown="True" "Pre-Spec. H(0)" {
              tunnel: [w710 w828] -> w619
              tunnel: w605 -> [_ w822]
              frame False {
                n233 = call-poly <vilib>:"Discrete Random.vi"("n"=360, "samples"=1) -> ("uniform (discrete) random data"=w723:i32[])  [unwired: 8 in, 1 out]
                n234 = Index Array(array=w723, index=0) -> (element=w718:i32)
                n235 = To Double Precision Float(number=w718) -> (double precision float=w717:dbl)
                n236 = Subtract(x=w717, y=180.0) -> (x-y=w720:dbl)
                n237 = Divide(x=w720, y=0.36) -> (x/y=w716:dbl)
                n238 = To Long Integer(number=w716) -> (32bit integer=w708:i32)
                n239 = Not Equal To 0?(x=w708) -> (x != 0?=w709:bool)
                n240 = To Double Precision Float(number=w708) -> (double precision float=w712:dbl)
                n241 = Greater Than 0?(x=w708) -> (x > 0?=w715:bool)
                n242 = Absolute Value(x=w708) -> (abs(x)=w714:i32)
                n243 = Multiply(x=0.36, y=w712) -> (x*y=w710:dbl)
                n244 = To Double Precision Float(number=w714) -> (double precision float=w713:dbl)
                n245 = case shown="True" w709 {
                  tunnel: w715 -> [_ w727]
                  tunnel: w713 -> [_ w726]
                  frame False {
                  }
                  frame True {
                    n246 = case shown="True" w727 {
                      tunnel: w726 -> [w728 w771]
                      frame True {
                        n247 = local read "Step Rate (Hz)"() -> (w731:dbl)
                        n248 = Reciprocal(x=w731) -> (1/x=w732:dbl)
                        n249 = node-c288(w732) -> (w734:T8)  [unwired: 3 in]
                        n250 = call-poly <vilib>:"DAQmx Create Virtual Channel.vi"("lines"=tag "Dev1/port0/line3") -> ("task out"=w730:refnum<k21>)  [unwired: 13 in, 1 out]
                        n251 = call-poly <vilib>:"DAQmx Create Virtual Channel.vi"("lines"=tag "Dev1/port0/line2") -> ("task out"=w729:refnum<k21>)  [unwired: 13 in, 1 out]
                        n252 = timed-loop {
                          timing: w734 -> [_]
                          timing-out: [_] -> w733
                          shift-right: [w747] -> _
                          shift-left: w730 -> [w745]
                          shift-right: [w746] -> _
                          shift-left: w729 -> [w744]
                          tunnel: w728 -> [w741]
                          i -> [w740]
                          stop <- w739 stop-if-true
                          n253 = node-c288() -> ()  [unwired: 1 in, 1 out]
                          n254 = flat-sequence {
                            tunnel: [w754] -> w749
                            tunnel: [w752] -> w748
                            tunnel: w745 -> [w751]
                            tunnel: w744 -> [w750]
                            tunnel: [w763] -> w747
                            tunnel: [w759] -> w746
                            tunnel: w749 -> [w762]
                            tunnel: w748 -> [w763]
                            frame #0 {
                              n255 = call-poly <vilib>:"DAQmx Write.vi"("task/channels in"=w751, "data"=FALSE) -> ("task out"=w753:refnum<k21>)  [unwired: 11 in, 2 out]
                              n256 = call-poly <vilib>:"DAQmx Write.vi"("task/channels in"=w750, "data"=TRUE) -> ("task out"=w755:refnum<k21>)  [unwired: 11 in, 2 out]
                              n257 = call <vilib>:"DAQmx Stop Task.vi"("task/channels in"=w753) -> ("task out"=w752:refnum<k21>)  [unwired: 13 in, 1 out]
                              n258 = call <vilib>:"DAQmx Stop Task.vi"("task/channels in"=w755) -> ("task out"=w754:refnum<k21>)  [unwired: 13 in, 1 out]
                            }
                            frame #1 {
                              n259 = call <vilib>:"DAQmx Start Task.vi"("task/channels in"=w762) -> ("task out"=w761:refnum<k21>)  [unwired: 13 in, 1 out]
                              n260 = call-poly <vilib>:"DAQmx Write.vi"("task/channels in"=w761, "data"=FALSE) -> ("task out"=w760:refnum<k21>)  [unwired: 11 in, 2 out]
                              n261 = call <vilib>:"DAQmx Stop Task.vi"("task/channels in"=w760) -> ("task out"=w759:refnum<k21>)  [unwired: 13 in, 1 out]
                            }
                          }
                          n262 = To Double Precision Float(number=w740) -> (double precision float=w742:dbl)
                          n263 = Increment(x=w742) -> (x+1=w743:dbl)
                          n264 = local read "Motor Error"() -> (w737:bool)
                          n265 = Equal?(x=w741, y=w743) -> (x = y?=w738:bool)
                          n266 = Or(x=w737, y=w738) -> (x .or. y?=w739:bool)
                          n267 = node-c288() -> ()  [unwired: 1 in, 1 out]
                        }
                        n268 = node-c288(w733) -> ()  [unwired: 1 out]
                      }
                      frame False {
                        n269 = local read "Step Rate (Hz)"() -> (w774:dbl)
                        n270 = Reciprocal(x=w774) -> (1/x=w775:dbl)
                        n271 = node-c288(w775) -> (w777:T8)  [unwired: 3 in]
                        n272 = call-poly <vilib>:"DAQmx Create Virtual Channel.vi"("lines"=tag "Dev1/port0/line3") -> ("task out"=w773:refnum<k21>)  [unwired: 13 in, 1 out]
                        n273 = call-poly <vilib>:"DAQmx Create Virtual Channel.vi"("lines"=tag "Dev1/port0/line2") -> ("task out"=w772:refnum<k21>)  [unwired: 13 in, 1 out]
                        n274 = timed-loop {
                          timing: w777 -> [_]
                          timing-out: [_] -> w776
                          shift-right: [w789] -> _
                          shift-left: w773 -> [w790]
                          shift-right: [w787] -> _
                          shift-left: w772 -> [w788]
                          tunnel: w771 -> [w783]
                          i -> [w782]
                          stop <- w781 stop-if-true
                          n275 = node-c288() -> ()  [unwired: 1 in, 1 out]
                          n276 = flat-sequence {
                            tunnel: [w797] -> w792
                            tunnel: [w795] -> w791
                            tunnel: w788 -> [w794]
                            tunnel: w790 -> [w793]
                            tunnel: [w806] -> w787
                            tunnel: [w802] -> w789
                            tunnel: w792 -> [w805]
                            tunnel: w791 -> [w806]
                            frame #0 {
                              n277 = call-poly <vilib>:"DAQmx Write.vi"("task/channels in"=w794, "data"=FALSE) -> ("task out"=w796:refnum<k21>)  [unwired: 11 in, 2 out]
                              n278 = call-poly <vilib>:"DAQmx Write.vi"("task/channels in"=w793, "data"=TRUE) -> ("task out"=w798:refnum<k21>)  [unwired: 11 in, 2 out]
                              n279 = call <vilib>:"DAQmx Stop Task.vi"("task/channels in"=w796) -> ("task out"=w795:refnum<k21>)  [unwired: 13 in, 1 out]
                              n280 = call <vilib>:"DAQmx Stop Task.vi"("task/channels in"=w798) -> ("task out"=w797:refnum<k21>)  [unwired: 13 in, 1 out]
                            }
                            frame #1 {
                              n281 = call <vilib>:"DAQmx Start Task.vi"("task/channels in"=w805) -> ("task out"=w804:refnum<k21>)  [unwired: 13 in, 1 out]
                              n282 = call-poly <vilib>:"DAQmx Write.vi"("task/channels in"=w804, "data"=FALSE) -> ("task out"=w803:refnum<k21>)  [unwired: 11 in, 2 out]
                              n283 = call <vilib>:"DAQmx Stop Task.vi"("task/channels in"=w803) -> ("task out"=w802:refnum<k21>)  [unwired: 13 in, 1 out]
                            }
                          }
                          n284 = To Double Precision Float(number=w782) -> (double precision float=w785:dbl)
                          n285 = Increment(x=w785) -> (x+1=w786:dbl)
                          n286 = Equal?(x=w783, y=w786) -> (x = y?=w784:bool)
                          n287 = local read "Motor Error"() -> (w780:bool)
                          n288 = Or(x=w780, y=w784) -> (x .or. y?=w781:bool)
                          n289 = node-c288() -> ()  [unwired: 1 in, 1 out]
                        }
                        n290 = node-c288(w776) -> ()  [unwired: 1 out]
                      }
                    }
                  }
                }
                n291 = local write "Heading (deg)"(w710) -> ()
                n292 = local write "H"(w710) -> ()
              }
              frame True {
                n293 = local read "Number of Trials"() -> (w818:i32)
                n294 = Subtract(x=w822, y=1) -> (x-y=w820:i32)
                n295 = Divide(x=w818, y=4) -> (x/y=w815:dbl)
                n296 = Divide(x=360.0, y=w815) -> (x/y=w814:dbl)
                n297 = Multiply(x=w814, y=w820) -> (x*y=w819:dbl)
                n298 = Subtract(x=180, y=w819) -> (x-y=w823:dbl)
                n299 = To Double Precision Float(number=w823) -> (double precision float=w825:dbl)
                n300 = Divide(x=w825, y=0.36) -> (x/y=w834:dbl)
                n301 = To Long Integer(number=w834) -> (32bit integer=w826:i32)
                n302 = Greater Than 0?(x=w826) -> (x > 0?=w833:bool)
                n303 = Not Equal To 0?(x=w826) -> (x != 0?=w827:bool)
                n304 = To Double Precision Float(number=w826) -> (double precision float=w830:dbl)
                n305 = Absolute Value(x=w826) -> (abs(x)=w832:i32)
                n306 = Multiply(x=0.36, y=w830) -> (x*y=w828:dbl)
                n307 = To Double Precision Float(number=w832) -> (double precision float=w831:dbl)
                n308 = case shown="True" w827 {
                  tunnel: w833 -> [_ w837]
                  tunnel: w831 -> [_ w836]
                  frame False {
                  }
                  frame True {
                    n309 = case shown="True" w837 {
                      tunnel: w836 -> [w838 w881]
                      frame True {
                        n310 = local read "Step Rate (Hz)"() -> (w841:dbl)
                        n311 = Reciprocal(x=w841) -> (1/x=w842:dbl)
                        n312 = node-c288(w842) -> (w844:T8)  [unwired: 3 in]
                        n313 = call-poly <vilib>:"DAQmx Create Virtual Channel.vi"("lines"=tag "Dev1/port0/line3") -> ("task out"=w840:refnum<k21>)  [unwired: 13 in, 1 out]
                        n314 = call-poly <vilib>:"DAQmx Create Virtual Channel.vi"("lines"=tag "Dev1/port0/line2") -> ("task out"=w839:refnum<k21>)  [unwired: 13 in, 1 out]
                        n315 = timed-loop {
                          timing: w844 -> [_]
                          timing-out: [_] -> w843
                          shift-right: [w857] -> _
                          shift-left: w840 -> [w855]
                          shift-right: [w856] -> _
                          shift-left: w839 -> [w854]
                          tunnel: w838 -> [w851]
                          i -> [w850]
                          stop <- w849 stop-if-true
                          n316 = node-c288() -> ()  [unwired: 1 in, 1 out]
                          n317 = flat-sequence {
                            tunnel: [w864] -> w859
                            tunnel: [w862] -> w858
                            tunnel: w855 -> [w861]
                            tunnel: w854 -> [w860]
                            tunnel: [w873] -> w857
                            tunnel: [w869] -> w856
                            tunnel: w859 -> [w872]
                            tunnel: w858 -> [w873]
                            frame #0 {
                              n318 = call-poly <vilib>:"DAQmx Write.vi"("task/channels in"=w861, "data"=FALSE) -> ("task out"=w863:refnum<k21>)  [unwired: 11 in, 2 out]
                              n319 = call-poly <vilib>:"DAQmx Write.vi"("task/channels in"=w860, "data"=TRUE) -> ("task out"=w865:refnum<k21>)  [unwired: 11 in, 2 out]
                              n320 = call <vilib>:"DAQmx Stop Task.vi"("task/channels in"=w863) -> ("task out"=w862:refnum<k21>)  [unwired: 13 in, 1 out]
                              n321 = call <vilib>:"DAQmx Stop Task.vi"("task/channels in"=w865) -> ("task out"=w864:refnum<k21>)  [unwired: 13 in, 1 out]
                            }
                            frame #1 {
                              n322 = call <vilib>:"DAQmx Start Task.vi"("task/channels in"=w872) -> ("task out"=w871:refnum<k21>)  [unwired: 13 in, 1 out]
                              n323 = call-poly <vilib>:"DAQmx Write.vi"("task/channels in"=w871, "data"=FALSE) -> ("task out"=w870:refnum<k21>)  [unwired: 11 in, 2 out]
                              n324 = call <vilib>:"DAQmx Stop Task.vi"("task/channels in"=w870) -> ("task out"=w869:refnum<k21>)  [unwired: 13 in, 1 out]
                            }
                          }
                          n325 = To Double Precision Float(number=w850) -> (double precision float=w852:dbl)
                          n326 = Increment(x=w852) -> (x+1=w853:dbl)
                          n327 = local read "Motor Error"() -> (w847:bool)
                          n328 = Equal?(x=w851, y=w853) -> (x = y?=w848:bool)
                          n329 = Or(x=w847, y=w848) -> (x .or. y?=w849:bool)
                          n330 = node-c288() -> ()  [unwired: 1 in, 1 out]
                        }
                        n331 = node-c288(w843) -> ()  [unwired: 1 out]
                      }
                      frame False {
                        n332 = local read "Step Rate (Hz)"() -> (w884:dbl)
                        n333 = Reciprocal(x=w884) -> (1/x=w885:dbl)
                        n334 = node-c288(w885) -> (w887:T8)  [unwired: 3 in]
                        n335 = call-poly <vilib>:"DAQmx Create Virtual Channel.vi"("lines"=tag "Dev1/port0/line3") -> ("task out"=w883:refnum<k21>)  [unwired: 13 in, 1 out]
                        n336 = call-poly <vilib>:"DAQmx Create Virtual Channel.vi"("lines"=tag "Dev1/port0/line2") -> ("task out"=w882:refnum<k21>)  [unwired: 13 in, 1 out]
                        n337 = timed-loop {
                          timing: w887 -> [_]
                          timing-out: [_] -> w886
                          shift-right: [w899] -> _
                          shift-left: w883 -> [w900]
                          shift-right: [w897] -> _
                          shift-left: w882 -> [w898]
                          tunnel: w881 -> [w893]
                          i -> [w892]
                          stop <- w891 stop-if-true
                          n338 = node-c288() -> ()  [unwired: 1 in, 1 out]
                          n339 = flat-sequence {
                            tunnel: [w907] -> w902
                            tunnel: [w905] -> w901
                            tunnel: w898 -> [w904]
                            tunnel: w900 -> [w903]
                            tunnel: [w916] -> w897
                            tunnel: [w912] -> w899
                            tunnel: w902 -> [w915]
                            tunnel: w901 -> [w916]
                            frame #0 {
                              n340 = call-poly <vilib>:"DAQmx Write.vi"("task/channels in"=w904, "data"=FALSE) -> ("task out"=w906:refnum<k21>)  [unwired: 11 in, 2 out]
                              n341 = call-poly <vilib>:"DAQmx Write.vi"("task/channels in"=w903, "data"=TRUE) -> ("task out"=w908:refnum<k21>)  [unwired: 11 in, 2 out]
                              n342 = call <vilib>:"DAQmx Stop Task.vi"("task/channels in"=w906) -> ("task out"=w905:refnum<k21>)  [unwired: 13 in, 1 out]
                              n343 = call <vilib>:"DAQmx Stop Task.vi"("task/channels in"=w908) -> ("task out"=w907:refnum<k21>)  [unwired: 13 in, 1 out]
                            }
                            frame #1 {
                              n344 = call <vilib>:"DAQmx Start Task.vi"("task/channels in"=w915) -> ("task out"=w914:refnum<k21>)  [unwired: 13 in, 1 out]
                              n345 = call-poly <vilib>:"DAQmx Write.vi"("task/channels in"=w914, "data"=FALSE) -> ("task out"=w913:refnum<k21>)  [unwired: 11 in, 2 out]
                              n346 = call <vilib>:"DAQmx Stop Task.vi"("task/channels in"=w913) -> ("task out"=w912:refnum<k21>)  [unwired: 13 in, 1 out]
                            }
                          }
                          n347 = To Double Precision Float(number=w892) -> (double precision float=w895:dbl)
                          n348 = Increment(x=w895) -> (x+1=w896:dbl)
                          n349 = Equal?(x=w893, y=w896) -> (x = y?=w894:bool)
                          n350 = local read "Motor Error"() -> (w890:bool)
                          n351 = Or(x=w890, y=w894) -> (x .or. y?=w891:bool)
                          n352 = node-c288() -> ()  [unwired: 1 in, 1 out]
                        }
                        n353 = node-c288(w886) -> ()  [unwired: 1 out]
                      }
                    }
                  }
                }
                n354 = local write "Heading (deg)"(w828) -> ()
                n355 = local write "H"(w828) -> ()
              }
            }
            n356 = flat-sequence {
              tunnel: w612 -> [w685]
              tunnel: [w685] -> w611
              tunnel: [w684] -> w610
              tunnel: w606 -> [w683]
              tunnel: w604 -> [w682]
              tunnel: [w682] -> w603
              tunnel: [w681] -> w602
              tunnel: w611 -> [w703]
              tunnel: w610 -> [w702]
              tunnel: [w701] -> w609
              tunnel: w603 -> [w700]
              tunnel: [w699] -> w601
              tunnel: w602 -> [w696]
              tunnel: w599 -> [w698]
              frame #0 {
                n357 = case shown="False" w683 {
                  tunnel: [w689 w695] -> w684
                  tunnel: [w686 w694] -> w681
                  frame False {
                    n358 = local read "Light Trial"() -> (w688:bool)
                    n359 = local read "Wind Trial"() -> (w687:bool)
                    n360 = case shown="True" w687 {
                      tunnel: [w690 w691] -> w686
                      frame False {
                        w690 = 0.0 ("Wind Intensity (V)")
                        n361 = local write "Wind Intensity (V)"(w690) -> ()
                      }
                      frame True {
                        w691 = 5.0 ("Wind Intensity (V)")
                        n362 = local write "Wind Intensity (V)"(w691) -> ()
                      }
                    }
                    n363 = case shown="True" w688 {
                      tunnel: [w692 w693] -> w689
                      frame False {
                        w692 = 0.0 ("Light Intensity (V)")
                        n364 = local write "Light Intensity (V)"(w692) -> ()
                      }
                      frame True {
                        w693 = 3.9 ("Light Intensity")
                        "Light Intensity (V)" <- w693
                      }
                    }
                  }
                  frame True {
                    n365 = local read "Light Intensity (V)"() -> (w695:dbl)
                    n366 = local read "Wind Intensity (V)"() -> (w694:dbl)
                  }
                }
              }
              frame #1 {
                n367 = Greater Than 0?(x=w696) -> (x > 0?=w697:bool)
                n368 = case shown="True" w697 {
                  tunnel: w698 -> [_ w707]
                  tunnel: w696 -> [_ w704]
                  frame False {
                  }
                  frame True {
                    n369 = call <vilib>:"DAQmx Start Task.vi"("task/channels in"=w707) -> ("task out"=w706:refnum<k21>)  [unwired: 13 in, 1 out]
                    n370 = call-poly <vilib>:"DAQmx Write.vi"("task/channels in"=w706, "data"=w704) -> ("task out"=w705:refnum<k21>)  [unwired: 11 in, 2 out]
                    n371 = call <vilib>:"DAQmx Stop Task.vi"("task/channels in"=w705) -> ()  [unwired: 13 in, 2 out]
                  }
                }
                n372 = Write to Binary File(file (use dialog)=w700, data=w696) -> (refnum out=w699:refnum<file>)  [unwired: 4 in, 2 out]
                n373 = Write to Binary File(file (use dialog)=w703, data=w702) -> (refnum out=w701:refnum<file>)  [unwired: 4 in, 2 out]
              }
            }
            n374 = call <vilib>:"Space Constant.vi"() -> ("String"=w650:string)
            n375 = call <vilib>:"Space Constant.vi"() -> ("String"=w670:string)
            n376 = call <vilib>:"Space Constant.vi"() -> ("String"=w637:string)
            n377 = call <vilib>:"Space Constant.vi"() -> ("String"=w661:string)
            n378 = Write to Binary File(file (use dialog)=w618, data=w617) -> (refnum out=w616:refnum<file>)  [unwired: 4 in, 2 out]
            n379 = call <vilib>:"Space Constant.vi"() -> ("String"=w627:string)
            n380 = Number To Fractional String(number=w623, precision (6)=i16 0) -> (F-format string=w653:string)  [unwired: 2 in]
            n381 = Number To Fractional String(number=w623, precision (6)=i16 0) -> (F-format string=w673:string)  [unwired: 2 in]
            n382 = Number To Fractional String(number=w623, precision (6)=i16 0) -> (F-format string=w640:string)  [unwired: 2 in]
            n383 = Number To Fractional String(number=w623, precision (6)=i16 0) -> (F-format string=w664:string)  [unwired: 2 in]
            n384 = Number To Fractional String(number=w623, precision (6)=i16 0) -> (F-format string=w630:string)  [unwired: 2 in]
            n385 = Concatenate Strings("trial", w650, w653, w650, "x_data") -> (w655:string)
            n386 = Concatenate Strings("trial", w670, w673, w670, "heading_data") -> (w675:string)
            n387 = Concatenate Strings("trial", w637, w640, w637, "LWBA_data") -> (w642:string)
            n388 = Concatenate Strings("trial", w661, w664, w661, "unfiltered deltaWBA") -> (w666:string)
            n389 = Concatenate Strings("trial", w627, w630, w627, "RWBA_data") -> (w632:string)
            n390 = local read "Wind Trial"() -> (w600:bool)
            n391 = String To Path(string=w655) -> (path=w656:path)
            n392 = String To Path(string=w675) -> (path=w676:path)
            n393 = String To Path(string=w642) -> (path=w643:path)
            n394 = String To Path(string=w666) -> (path=w667:path)
            n395 = String To Path(string=w632) -> (path=w633:path)
            n396 = Build Path(base path=w624, name or relative path=w656) -> (appended path=w649:path)
            n397 = Build Path(base path=w624, name or relative path=w676) -> (appended path=w669:path)
            n398 = Build Path(base path=w624, name or relative path=w643) -> (appended path=w636:path)
            n399 = Build Path(base path=w624, name or relative path=w667) -> (appended path=w660:path)
            n400 = Build Path(base path=w624, name or relative path=w633) -> (appended path=w626:path)
            n401 = Boolean To (0,1)(Boolean=w600) -> (0, 1=w614:i16)
            n402 = Open/Create/Replace File(file path (use dialog)=w649, operation (0:open)=T4."create", access (0:read/write)=enum16{"read/write", "read-only", "write-only"}."write-only") -> (refnum out=w647:refnum<file>)  [unwired: 3 in, 2 out]
            n403 = Open/Create/Replace File(file path (use dialog)=w669, operation (0:open)=T4."create", access (0:read/write)=enum16{"read/write", "read-only", "write-only"}."write-only") -> (refnum out=w646:refnum<file>)  [unwired: 3 in, 2 out]
            n404 = Open/Create/Replace File(file path (use dialog)=w636, operation (0:open)=T4."create", access (0:read/write)=enum16{"read/write", "read-only", "write-only"}."write-only") -> (refnum out=w622:refnum<file>)  [unwired: 3 in, 2 out]
            n405 = Open/Create/Replace File(file path (use dialog)=w660, operation (0:open)=T4."create", access (0:read/write)=enum16{"read/write", "read-only", "write-only"}."write-only") -> (refnum out=w645:refnum<file>)  [unwired: 3 in, 2 out]
            n406 = Open/Create/Replace File(file path (use dialog)=w626, operation (0:open)=T4."create", access (0:read/write)=enum16{"read/write", "read-only", "write-only"}."write-only") -> (refnum out=w621:refnum<file>)  [unwired: 3 in, 2 out]
            n407 = Write to Binary File(file (use dialog)=w615, data=w614) -> (refnum out=w613:refnum<file>)  [unwired: 4 in, 2 out]
          }
          frame #3 {
            n408 = call-poly <vilib>:"DAQmx Create Virtual Channel.vi"("lines"=tag "Dev1/port0/line7") -> ("task out"=w953:refnum<k21>)  [unwired: 13 in, 1 out]
            n409 = call-poly <vilib>:"DAQmx Create Virtual Channel.vi"("lines"=tag "Dev1/port0/line3") -> ("task out"=w941:refnum<k21>)  [unwired: 13 in, 1 out]
            n410 = call-poly <vilib>:"DAQmx Create Virtual Channel.vi"("lines"=tag "Dev1/port0/line2") -> ("task out"=w942:refnum<k21>)  [unwired: 13 in, 1 out]
            n411 = call-poly <vilib>:"DAQmx Create Virtual Channel.vi"("lines"=tag "Dev1/port0/line6") -> ("task out"=w934:refnum<k21>)  [unwired: 13 in, 1 out]
            n412 = call-poly <vilib>:"DAQmx Create Virtual Channel.vi"("physical channels"=tag "Dev1/ao0") -> ("task out"=w929:refnum<k21>)  [unwired: 13 in, 1 out]
            n413 = Reciprocal(x="Data Rate (Hz)") -> (1/x=w961:dbl)
            n414 = call-poly <vilib>:"DAQmx Create Virtual Channel.vi"("lines"=tag "Dev1/port0/line1") -> ("task out"=w937:refnum<k21>)  [unwired: 13 in, 1 out]
            n415 = node-c288(w961) -> (w963:T8)  [unwired: 3 in]
            n416 = timed-loop {
              timing: w963 -> [_]
              timing-out: [_] -> w962
              tunnel: w959 -> [w1054]
              tunnel: w958 -> [w1055]
              tunnel: w957 -> [w1053]
              shift-right: [w1034] -> w951
              shift-left: w942 -> [w1036]
              shift-right: [w1035] -> w952
              shift-left: w941 -> [w1037]
              tunnel: w956 -> [w1052]
              tunnel: [w1051] -> w955
              shift-right: [w1049] -> _
              shift-left: w953 -> [w1050]
              shift-right: [w1046] -> _
              shift-left: w936 -> [w1047]
              tunnel: w950 -> [w1045]
              tunnel: [w1044] -> w949
              tunnel: [w1043] -> w948
              tunnel: w947 -> [w1042]
              tunnel: w946 -> [w1041]
              tunnel: w945 -> [w1040]
              tunnel: [w1039] -> w944
              tunnel: [w1038] -> w943
              shift-right: [w1030] -> _
              shift-left: w937 -> [w1033]
              shift-right: [w975] -> _
              shift-left: _ -> [w983]
              shift-right: [w977] -> w933
              shift-left: w934 -> [w980]
              shift-right: [w965] -> w927
              shift-left: w929 -> [w967]
              i -> [w1048]
              stop <- w1027 stop-if-true
              w1016 = T13 {"Search Direction"=0, "Edge Options"={"Edge Polarity"=0, "Kernel Size"=3, "Width"=3, "Minimum Edge Strength"=2.0, "Interpolation Type"=enum."Bilinear Fixed", "Data Processing Method"=enum."Average"}, "Show Search Area"=TRUE, "Show Search Lines"=TRUE, "Show Edges Found"=TRUE, "Show Result"=TRUE, "Search Area Color"=65280, "Search Lines Color"=255, "Edge Locations Color"=16776960, "Result Color"=16711680, "Overlay Group Name"=""} ("Options")
              n417 = node-c288() -> ()  [unwired: 1 in, 1 out]
              n418 = To Double Precision Float(number=w1048) -> (double precision float=w987:dbl)
              n419 = local read "Wind Trial"() -> (w964:bool)
              n420 = local read "Light Intensity (V)"() -> (w966:dbl)
              n421 = local read "Data Rate (Hz)"() -> (w1004:dbl)
              n422 = Increment(x=w987) -> (x+1=w998:dbl)
              n423 = call <vilib>:"DAQmx Start Task.vi"("task/channels in"=w967) -> ("task out"=w969:refnum<k21>)  [unwired: 13 in, 1 out]
              n424 = call <vilib>:"DAQmx Start Task.vi"("task/channels in"=w980) -> ("task out"=w979:refnum<k21>)  [unwired: 13 in, 1 out]
              n425 = call <vilib>:"DAQmx Start Task.vi"("task/channels in"=w1050) -> ("task out"=w1007:refnum<k21>)  [unwired: 13 in, 1 out]
              n426 = call <vilib>:"DAQmx Start Task.vi"("task/channels in"=w1033) -> ("task out"=w1032:refnum<k21>)  [unwired: 13 in, 1 out]
              n427 = Divide(x=w998, y=w1004) -> (x/y=w1001:dbl)
              n428 = call-poly <vilib>:"DAQmx Write.vi"("task/channels in"=w969, "data"=w966) -> ("task out"=w968:refnum<k21>)  [unwired: 11 in, 2 out]
              n429 = call-poly <vilib>:"DAQmx Write.vi"("task/channels in"=w979, "data"=w964) -> ("task out"=w978:refnum<k21>)  [unwired: 11 in, 2 out]
              n430 = local read "Odor Duration (s)"() -> (w981:dbl)
              "Odor Duration (s)" <- w981
              n431 = call "IMAQ Create"("Image Name"="flyim") -> ("New Image"=w1026:T3)  [unwired: 3 in, 2 out]
              n432 = Greater?(x=w1001, y="Trial Duration (s)") -> (0:→"Trial End":bool)
              n433 = call <vilib>:"DAQmx Stop Task.vi"("task/channels in"=w968) -> ("task out"=w965:refnum<k21>)  [unwired: 13 in, 1 out]
              n434 = call <vilib>:"DAQmx Stop Task.vi"("task/channels in"=w978) -> ("task out"=w977:refnum<k21>)  [unwired: 13 in, 1 out]
              n435 = call-poly <vilib>:"DAQmx Read.vi"("task/channels in"=w1032) -> ("task out"=w1031:refnum<k21>, "data"=→"Motor Error":bool)  [unwired: 12 in, 1 out]
              n436 = call <vilib>:"IMAQdx Grab.vi"("Wait for Next Buffer? (Yes)"=FALSE, "Image In"=w1026, "Session In"=w1055) -> ("Image Out"=w1017:T3)  [unwired: 1 in, 7 out]
              n437 = call "IMAQ Threshold"("Keep/Replace Value (Replace)"=FALSE, "Range"="Image Threshold", "Image Src"=w1017) -> ("Image Dst Out"=w1022:T3)  [unwired: 7 in, 1 out]
              n438 = Add(x="Odor Onset Time (s)", y=w981) -> (x+y=w1003:dbl)
              n439 = call <vilib>:"DAQmx Stop Task.vi"("task/channels in"=w1031) -> ("task out"=w1030:refnum<k21>)  [unwired: 13 in, 1 out]
              n440 = call "IMAQ Find Edge"("Line Fit Options"="L options", "Options"=w1016, "ROI Descriptor"=w1054, "Image"=w1022) -> ("Straight Edges"=w1019:T14, "Image Out"=w1021:T3)  [unwired: 4 in, 2 out]
              n441 = call "IMAQ Find Edge"("Line Fit Options"="R options", "Options"=w1016, "ROI Descriptor"=w1053, "Image"=w1021) -> ("Straight Edges"=w1018:T14, "Image Out"=→"Image":T3)  [unwired: 4 in, 2 out]
              n442 = In Range and Coerce(upper limit=w1003, x=w1001, lower limit="Odor Onset Time (s)") -> (In Range?=w1005:bool)  [unwired: 1 out]
              "Odor On" <- w1005
              n443 = Array To Cluster(array=w1018) -> (cluster=w1009:T15)
              n444 = Array To Cluster(array=w1019) -> (cluster=w1008:T15)
              n445 = call-poly <vilib>:"DAQmx Write.vi"("task/channels in"=w1007, "data"=w1005) -> ("task out"=w1006:refnum<k21>)  [unwired: 11 in, 2 out]
              n446 = Unbundle By Name(w1009) -> ("Straight Edges[0].Angle (Pixel)"=w1014:dbl)
              n447 = Unbundle By Name(w1008) -> ("Straight Edges[0].Angle (Pixel)"=w1015:dbl)
              n448 = call <vilib>:"DAQmx Stop Task.vi"("task/channels in"=w1006) -> ("task out"=w1049:refnum<k21>)  [unwired: 13 in, 1 out]
              n449 = Absolute Value(x=w1014) -> (abs(x)=w988:dbl)
              "L WBA" <- w988
              n450 = Absolute Value(x=w1015) -> (abs(x)=w989:dbl)
              "R WBA" <- w989
              n451 = Write to Binary File(file (use dialog)=w1040, data=w989) -> (refnum out=w1039:refnum<file>)  [unwired: 4 in, 2 out]
              n452 = Write to Binary File(file (use dialog)=w1041, data=w988) -> (refnum out=w1038:refnum<file>)  [unwired: 4 in, 2 out]
              n453 = Subtract(x=w988, y=w989) -> (x-y=w1012:dbl)
              "L-R WBA" <- w1012
              n454 = case shown="False" "Reversed Tether?" {
                tunnel: w1012 -> [w1058 w1060]
                tunnel: [w1057 w1059] -> w1011
                tunnel: "L-R WBA Offset (deg)" -> [w1056 w1061]
                frame False {
                  n455 = Add ("Add.vi")(x=w1058, y=w1056) -> (x+y=w1057:dbl)
                }
                frame True {
                  n456 = Subtract(x=w1060, y=w1061) -> (x-y=w1059:dbl)
                }
              }
              n457 = Multiply(x=w1011, y="deltaWBA Scale Factor (k, unitless)") -> (x*y=w1013:dbl)
              n458 = case shown="False" "Reversed Tether?" {
                tunnel: w1013 -> [w1063 w1064]
                tunnel: [w1062 w1064] -> w973
                frame False {
                  n459 = Negate(x=w1063) -> (-x=w1062:dbl)
                }
                frame True {
                }
              }
              "Scaled deltaWBA (deg)" <- w973
              "deltaWBA" <- w973
              n460 = Greater Or Equal To 0?(x=w973) -> (x >= 0?=w974:bool)
              n461 = case shown="False" w974 {
                tunnel: [w1075 w1092] -> w975
                tunnel: "Max steps/sample" -> [w1074 w1088]
                tunnel: w973 -> [w1068 w1087]
                frame False {
                  n462 = Absolute Value(x=w1068) -> (abs(x)=w1069:dbl)
                  n463 = Quotient & Remainder(x=w1069, y=0.36) -> (x-y*floor(x/y)=w1067:dbl, floor(x/y)=w1070:dbl)
                  n464 = Greater?(x=w1067, y=0.18) -> (0:w1071:bool)
                  n465 = Negate(x=w1074) -> (-x=w1076:dbl)
                  n466 = case shown="True" w1071 {
                    tunnel: w1070 -> [w1078 w1081]
                    tunnel: [w1078 w1079] -> w1066
                    frame False {
                    }
                    frame True {
                      n467 = Add(x=w1081, y=1.0) -> (x+y=w1079:dbl)
                    }
                  }
                  n468 = Negate(x=w1066) -> (-x=w1065:dbl)
                  n469 = Less?(x=w1065, y=w1076) -> (x < y?=w1077:bool)
                  n470 = case shown="False" w1077 {
                    tunnel: w1076 -> [_ w1083]
                    tunnel: [w1082 w1083] -> w1075
                    tunnel: w1065 -> [w1082 _]
                    frame False {
                    }
                    frame True {
                    }
                  }
                }
                frame True {
                  n471 = Quotient & Remainder(x=w1087, y=0.36) -> (x-y*floor(x/y)=w1085:dbl, floor(x/y)=w1090:dbl)
                  n472 = Greater?(x=w1085, y=0.18) -> (0:w1086:bool)
                  n473 = case shown="True" w1086 {
                    tunnel: w1090 -> [w1094 w1097]
                    tunnel: [w1094 w1095] -> w1091
                    frame False {
                    }
                    frame True {
                      n474 = Add(x=w1097, y=1.0) -> (x+y=w1095:dbl)
                    }
                  }
                  n475 = Greater?(x=w1091, y=w1088) -> (0:w1093:bool)
                  n476 = case shown="False" w1093 {
                    tunnel: w1088 -> [_ w1099]
                    tunnel: [w1098 w1099] -> w1092
                    tunnel: w1091 -> [w1098 _]
                    frame False {
                    }
                    frame True {
                    }
                  }
                }
              }
              "X (steps/sample)" <- w975
              "X (steps/sample)" <- w975
              n477 = Multiply(x=0.36 ("y"), y=w975) -> (x*y=w990:dbl)
              n478 = Add ("Add.vi")(x=w990, y=w1047) -> (x+y=w994:dbl)
              n479 = Add(x=w994, y=180.0 ("x")) -> (x+y=w995:dbl)
              n480 = Quotient & Remainder(x=w995, y=360.0) -> (x-y*floor(x/y)=w996:dbl)  [unwired: 1 out]
              n481 = Subtract(x=w996, y=180.0) -> (x-y=w1046:dbl)
              "H" <- w1046
              "Heading (deg)" <- w1046
              n482 = Write to Binary File(file (use dialog)=w1045, data=w1046) -> (refnum out=w1044:refnum<file>)  [unwired: 4 in, 2 out]
              n483 = Write to Binary File(file (use dialog)=w1042, data=w973) -> (refnum out=w1051:refnum<file>)  [unwired: 4 in, 2 out]
              n484 = Write to Binary File(file (use dialog)=w1052, data=w975) -> (refnum out=w1043:refnum<file>)  [unwired: 4 in, 2 out]
              n485 = Not Equal To 0?(x=w983) -> (x != 0?=w984:bool)
              n486 = case shown="True" w984 {
                tunnel: w1037 -> [w1101 w1108]
                tunnel: w1036 -> [w1100 w1107]
                tunnel: w983 -> [_ w1106]
                tunnel: [w1100 w1105] -> w1034
                tunnel: [w1101 w1104] -> w1035
                frame False {
                }
                frame True {
                  n487 = Reciprocal(x="Step Rate (Hz)") -> (1/x=w1102:dbl)
                  n488 = node-c288(w1102) -> (w1110:T8)  [unwired: 3 in]
                  n489 = timed-loop {
                    timing: w1110 -> [_]
                    timing-out: [_] -> w1109
                    tunnel: w1106 -> [w1124]
                    shift-right: [w1117] -> w1104
                    shift-left: w1108 -> [w1121]
                    shift-right: [w1116] -> w1105
                    shift-left: w1107 -> [w1119]
                    i -> [w1115]
                    stop <- w1113 stop-if-true
                    n490 = node-c288() -> ()  [unwired: 1 in, 1 out]
                    n491 = To Double Precision Float(number=w1115) -> (double precision float=w1114:dbl)
                    n492 = Absolute Value(x=w1124) -> (abs(x)=w1123:dbl)
                    n493 = call <vilib>:"DAQmx Start Task.vi"("task/channels in"=w1121) -> ("task out"=w1120:refnum<k21>)  [unwired: 13 in, 1 out]
                    n494 = call <vilib>:"DAQmx Start Task.vi"("task/channels in"=w1119) -> ("task out"=w1118:refnum<k21>)  [unwired: 13 in, 1 out]
                    n495 = Increment(x=w1114) -> (x+1=w1122:dbl)
                    n496 = Greater Than 0?(x=w1124) -> (x > 0?=w1125:bool)
                    n497 = Equal?(x=w1123, y=w1122) -> (x = y?=w1112:bool)
                    n498 = case shown="False" w1125 {
                      tunnel: [w1128 w1148] -> w1117
                      tunnel: [w1129 w1149] -> w1116
                      tunnel: w1118 -> [w1131 w1151]
                      tunnel: w1120 -> [w1130 w1150]
                      frame True {
                        n499 = flat-sequence {
                          tunnel: w1131 -> [w1139]
                          tunnel: w1130 -> [w1138]
                          tunnel: [w1134] -> w1127
                          tunnel: [w1132] -> w1126
                          tunnel: [w1145] -> w1128
                          tunnel: [w1141] -> w1129
                          tunnel: w1127 -> [w1144]
                          tunnel: w1126 -> [w1145]
                          frame #0 {
                            n500 = call-poly <vilib>:"DAQmx Write.vi"("task/channels in"=w1138, "data"=FALSE) -> ("task out"=w1133:refnum<k21>)  [unwired: 11 in, 2 out]
                            n501 = call-poly <vilib>:"DAQmx Write.vi"("task/channels in"=w1139, "data"=TRUE) -> ("task out"=w1135:refnum<k21>)  [unwired: 11 in, 2 out]
                            n502 = call <vilib>:"DAQmx Stop Task.vi"("task/channels in"=w1133) -> ("task out"=w1132:refnum<k21>)  [unwired: 13 in, 1 out]
                            n503 = call <vilib>:"DAQmx Stop Task.vi"("task/channels in"=w1135) -> ("task out"=w1134:refnum<k21>)  [unwired: 13 in, 1 out]
                          }
                          frame #1 {
                            n504 = call <vilib>:"DAQmx Start Task.vi"("task/channels in"=w1144) -> ("task out"=w1143:refnum<k21>)  [unwired: 13 in, 1 out]
                            n505 = call-poly <vilib>:"DAQmx Write.vi"("task/channels in"=w1143, "data"=FALSE) -> ("task out"=w1142:refnum<k21>)  [unwired: 11 in, 2 out]
                            n506 = call <vilib>:"DAQmx Stop Task.vi"("task/channels in"=w1142) -> ("task out"=w1141:refnum<k21>)  [unwired: 13 in, 1 out]
                          }
                        }
                      }
                      frame False {
                        n507 = flat-sequence {
                          tunnel: w1151 -> [w1159]
                          tunnel: w1150 -> [w1158]
                          tunnel: [w1154] -> w1147
                          tunnel: [w1152] -> w1146
                          tunnel: [w1161] -> w1148
                          tunnel: [w1160] -> w1149
                          tunnel: w1147 -> [w1160]
                          tunnel: w1146 -> [w1162]
                          frame #0 {
                            n508 = call-poly <vilib>:"DAQmx Write.vi"("task/channels in"=w1158, "data"=TRUE) -> ("task out"=w1153:refnum<k21>)  [unwired: 11 in, 2 out]
                            n509 = call-poly <vilib>:"DAQmx Write.vi"("task/channels in"=w1159, "data"=FALSE) -> ("task out"=w1155:refnum<k21>)  [unwired: 11 in, 2 out]
                            n510 = call <vilib>:"DAQmx Stop Task.vi"("task/channels in"=w1153) -> ("task out"=w1152:refnum<k21>)  [unwired: 13 in, 1 out]
                            n511 = call <vilib>:"DAQmx Stop Task.vi"("task/channels in"=w1155) -> ("task out"=w1154:refnum<k21>)  [unwired: 13 in, 1 out]
                          }
                          frame #1 {
                            n512 = call <vilib>:"DAQmx Start Task.vi"("task/channels in"=w1162) -> ("task out"=w1165:refnum<k21>)  [unwired: 13 in, 1 out]
                            n513 = call-poly <vilib>:"DAQmx Write.vi"("task/channels in"=w1165, "data"=FALSE) -> ("task out"=w1164:refnum<k21>)  [unwired: 11 in, 2 out]
                            n514 = call <vilib>:"DAQmx Stop Task.vi"("task/channels in"=w1164) -> ("task out"=w1161:refnum<k21>)  [unwired: 13 in, 1 out]
                          }
                        }
                      }
                    }
                    n515 = local read "Motor Error"() -> (w1111:bool)
                    n516 = Or(x=w1112, y=w1111) -> (x .or. y?=w1113:bool)
                    n517 = node-c288() -> ()  [unwired: 1 in, 1 out]
                  }
                  n518 = node-c288(w1109) -> ()  [unwired: 1 out]
                }
              }
              n519 = local read "Motor Error"() -> (w1028:bool)
              n520 = local read "Trial End"() -> (w1029:bool)
              n521 = Or(x=w1029, y=w1028) -> (x .or. y?=w1027:bool)
              n522 = node-c288() -> ()  [unwired: 1 in, 1 out]
            }
            n523 = node-c288(w962) -> ()  [unwired: 1 out]
          }
          frame #4 {
            n524 = local read "H"() -> (w1190:dbl)
            n525 = Absolute Value(x=w1190) -> (abs(x)=w1182:dbl)
            n526 = Close File(refnum=w1202) -> ()  [unwired: 1 in, 2 out]
            n527 = Close File(refnum=w1201) -> ()  [unwired: 1 in, 2 out]
            n528 = Close File(refnum=w1200) -> ()  [unwired: 1 in, 2 out]
            n529 = Close File(refnum=w1199) -> ()  [unwired: 1 in, 2 out]
            n530 = Close File(refnum=w1203) -> ()  [unwired: 1 in, 2 out]
            n531 = Greater Than 0?(x=w1190) -> (x > 0?=w1198:bool)
            n532 = To Long Integer(number=w1182) -> (32bit integer=w1181:i32)
            n533 = Not Equal To 0?(x=w1181) -> (x != 0?=w1197:bool)
            n534 = case shown="True" w1197 {
              tunnel: w1205 -> [_ w1209]
              tunnel: w1204 -> [_ w1208]
              tunnel: w1198 -> [_ w1207]
              tunnel: w1190 -> [_ w1206]
              frame False {
              }
              frame True {
                n535 = case shown="False" w1207 {
                  tunnel: w1209 -> [w1218 w1267]
                  tunnel: w1208 -> [w1217 w1266]
                  tunnel: w1206 -> [w1215 w1264]
                  frame True {
                    n536 = local read "X (steps/sample)"() -> (w1213:dbl)
                    n537 = Divide(x=w1215, y=0.36) -> (x/y=w1210:dbl)
                    n538 = Subtract(x=w1210, y=w1213) -> (x-y=w1212:dbl)
                    n539 = local read "Step Rate (Hz)"() -> (w1216:dbl)
                    n540 = Reciprocal(x=w1216) -> (1/x=w1219:dbl)
                    n541 = node-c288(w1219) -> (w1221:T8)  [unwired: 3 in]
                    n542 = Absolute Value(x=w1212) -> (abs(x)=w1211:dbl)
                    n543 = timed-loop {
                      timing: w1221 -> [_]
                      timing-out: [_] -> w1220
                      shift-right: [w1233] -> _
                      shift-left: w1217 -> [w1231]
                      shift-right: [w1234] -> _
                      shift-left: w1218 -> [w1232]
                      tunnel: w1211 -> [w1225]
                      i -> [w1223]
                      stop <- w1228 stop-if-true
                      n544 = node-c288() -> ()  [unwired: 1 in, 1 out]
                      n545 = To Long Integer(number=w1223) -> (32bit integer=w1222:i32)
                      n546 = To Long Integer(number=w1225) -> (32bit integer=w1224:i32)
                      n547 = flat-sequence {
                        tunnel: w1232 -> [w1241]
                        tunnel: w1231 -> [w1239]
                        tunnel: [w1244] -> w1230
                        tunnel: [w1242] -> w1229
                        tunnel: [w1251] -> w1233
                        tunnel: [w1246] -> w1234
                        tunnel: w1230 -> [w1249]
                        tunnel: w1229 -> [w1251]
                        frame #0 {
                          n548 = call <vilib>:"DAQmx Start Task.vi"("task/channels in"=w1241) -> ("task out"=w1240:refnum<k21>)  [unwired: 13 in, 1 out]
                          n549 = call <vilib>:"DAQmx Start Task.vi"("task/channels in"=w1239) -> ("task out"=w1238:refnum<k21>)  [unwired: 13 in, 1 out]
                          n550 = call-poly <vilib>:"DAQmx Write.vi"("task/channels in"=w1240, "data"=TRUE) -> ("task out"=w1245:refnum<k21>)  [unwired: 11 in, 2 out]
                          n551 = call-poly <vilib>:"DAQmx Write.vi"("task/channels in"=w1238, "data"=FALSE) -> ("task out"=w1243:refnum<k21>)  [unwired: 11 in, 2 out]
                          n552 = call <vilib>:"DAQmx Stop Task.vi"("task/channels in"=w1245) -> ("task out"=w1244:refnum<k21>)  [unwired: 13 in, 1 out]
                          n553 = call <vilib>:"DAQmx Stop Task.vi"("task/channels in"=w1243) -> ("task out"=w1242:refnum<k21>)  [unwired: 13 in, 1 out]
                        }
                        frame #1 {
                          n554 = call <vilib>:"DAQmx Start Task.vi"("task/channels in"=w1249) -> ("task out"=w1248:refnum<k21>)  [unwired: 13 in, 1 out]
                          n555 = call-poly <vilib>:"DAQmx Write.vi"("task/channels in"=w1248, "data"=FALSE) -> ("task out"=w1247:refnum<k21>)  [unwired: 11 in, 2 out]
                          n556 = call <vilib>:"DAQmx Stop Task.vi"("task/channels in"=w1247) -> ("task out"=w1246:refnum<k21>)  [unwired: 13 in, 1 out]
                        }
                      }
                      n557 = Increment(x=w1222) -> (x+1=w1235:i32)
                      n558 = Equal?(x=w1224, y=w1235) -> (x = y?=w1226:bool)
                      n559 = local read "Motor Error"() -> (w1227:bool)
                      n560 = Or(x=w1227, y=w1226) -> (x .or. y?=w1228:bool)
                      n561 = node-c288() -> ()  [unwired: 1 in, 1 out]
                    }
                    n562 = node-c288(w1220) -> ()  [unwired: 1 out]
                  }
                  frame False {
                    n563 = local read "X (steps/sample)"() -> (w1261:dbl)
                    n564 = Divide(x=w1264, y=0.36) -> (x/y=w1262:dbl)
                    n565 = local read "Step Rate (Hz)"() -> (w1265:dbl)
                    n566 = Reciprocal(x=w1265) -> (1/x=w1268:dbl)
                    n567 = node-c288(w1268) -> (w1270:T8)  [unwired: 3 in]
                    n568 = Subtract(x=w1262, y=w1261) -> (x-y=w1260:dbl)
                    n569 = Absolute Value(x=w1260) -> (abs(x)=w1259:dbl)
                    n570 = timed-loop {
                      timing: w1270 -> [_]
                      timing-out: [_] -> w1269
                      shift-right: [w1282] -> _
                      shift-left: w1266 -> [w1280]
                      shift-right: [w1283] -> _
                      shift-left: w1267 -> [w1281]
                      tunnel: w1259 -> [w1272]
                      i -> [w1274]
                      stop <- w1277 stop-if-true
                      n571 = node-c288() -> ()  [unwired: 1 in, 1 out]
                      n572 = To Long Integer(number=w1272) -> (32bit integer=w1271:i32)
                      n573 = To Long Integer(number=w1274) -> (32bit integer=w1273:i32)
                      n574 = flat-sequence {
                        tunnel: w1281 -> [w1290]
                        tunnel: w1280 -> [w1288]
                        tunnel: [w1293] -> w1279
                        tunnel: [w1291] -> w1278
                        tunnel: [w1296] -> w1282
                        tunnel: [w1295] -> w1283
                        tunnel: w1279 -> [w1295]
                        tunnel: w1278 -> [w1297]
                        frame #0 {
                          n575 = call <vilib>:"DAQmx Start Task.vi"("task/channels in"=w1290) -> ("task out"=w1289:refnum<k21>)  [unwired: 13 in, 1 out]
                          n576 = call <vilib>:"DAQmx Start Task.vi"("task/channels in"=w1288) -> ("task out"=w1287:refnum<k21>)  [unwired: 13 in, 1 out]
                          n577 = call-poly <vilib>:"DAQmx Write.vi"("task/channels in"=w1289, "data"=FALSE) -> ("task out"=w1294:refnum<k21>)  [unwired: 11 in, 2 out]
                          n578 = call-poly <vilib>:"DAQmx Write.vi"("task/channels in"=w1287, "data"=TRUE) -> ("task out"=w1292:refnum<k21>)  [unwired: 11 in, 2 out]
                          n579 = call <vilib>:"DAQmx Stop Task.vi"("task/channels in"=w1294) -> ("task out"=w1293:refnum<k21>)  [unwired: 13 in, 1 out]
                          n580 = call <vilib>:"DAQmx Stop Task.vi"("task/channels in"=w1292) -> ("task out"=w1291:refnum<k21>)  [unwired: 13 in, 1 out]
                        }
                        frame #1 {
                          n581 = call <vilib>:"DAQmx Start Task.vi"("task/channels in"=w1297) -> ("task out"=w1299:refnum<k21>)  [unwired: 13 in, 1 out]
                          n582 = call-poly <vilib>:"DAQmx Write.vi"("task/channels in"=w1299, "data"=FALSE) -> ("task out"=w1298:refnum<k21>)  [unwired: 11 in, 2 out]
                          n583 = call <vilib>:"DAQmx Stop Task.vi"("task/channels in"=w1298) -> ("task out"=w1296:refnum<k21>)  [unwired: 13 in, 1 out]
                        }
                      }
                      n584 = Increment(x=w1273) -> (x+1=w1284:i32)
                      n585 = Equal?(x=w1271, y=w1284) -> (x = y?=w1276:bool)
                      n586 = local read "Motor Error"() -> (w1275:bool)
                      n587 = Or(x=w1275, y=w1276) -> (x .or. y?=w1277:bool)
                      n588 = node-c288() -> ()  [unwired: 1 in, 1 out]
                    }
                    n589 = node-c288(w1269) -> ()  [unwired: 1 out]
                  }
                }
              }
            }
            n590 = call <vilib>:"DAQmx Start Task.vi"("task/channels in"=w1186) -> ("task out"=w1188:refnum<k21>)  [unwired: 13 in, 1 out]
            n591 = call <vilib>:"DAQmx Start Task.vi"("task/channels in"=w1194) -> ("task out"=w1193:refnum<k21>)  [unwired: 13 in, 1 out]
            n592 = call-poly <vilib>:"DAQmx Write.vi"("task/channels in"=w1188, "data"=0.0) -> ("task out"=w1187:refnum<k21>)  [unwired: 11 in, 2 out]
            n593 = call-poly <vilib>:"DAQmx Write.vi"("task/channels in"=w1193, "data"=FALSE) -> ("task out"=w1192:refnum<k21>)  [unwired: 11 in, 2 out]
            n594 = call <vilib>:"DAQmx Stop Task.vi"("task/channels in"=w1187) -> ()  [unwired: 13 in, 2 out]
            n595 = call <vilib>:"DAQmx Stop Task.vi"("task/channels in"=w1192) -> ()  [unwired: 13 in, 2 out]
          }
          frame #5 {
            n596 = Greater Than 0?(x=w1309) -> (x > 0?=w1310:bool)
            n597 = case shown="True" w1310 {
              tunnel: w1315 -> [w1328 w1340]
              tunnel: w1309 -> [_ w1333]
              tunnel: [w1327 w1332] -> w1314
              tunnel: [w1326 w1331] -> w1313
              tunnel: [w1324 w1330] -> w1312
              tunnel: [w1325 w1329] -> w1311
              frame False {
                n598 = Unbundle(w1328) -> ("y"=w1327:i32, "y"=w1326:i32, "y"=w1324:i32, "y"=w1325:i32)
              }
              frame True {
                n599 = Unbundle(w1340) -> ("y"=w1337:i32, "y"=w1336:i32, "y"=w1335:i32, "y"=w1334:i32)
                n600 = Greater?(x=w1333, y=2.0) -> (0:w1338:bool)
                n601 = case shown="True" w1338 {
                  tunnel: w1337 -> [w1348 w1369]
                  tunnel: w1336 -> [w1347 w1368]
                  tunnel: w1335 -> [w1346 w1367]
                  tunnel: w1334 -> [w1345 w1366]
                  tunnel: w1333 -> [w1349 w1371]
                  tunnel: [w1344 w1362] -> w1332
                  tunnel: [w1343 w1363] -> w1331
                  tunnel: [w1342 w1365] -> w1330
                  tunnel: [w1341 w1364] -> w1329
                  frame False {
                    n602 = Greater?(x=w1349, y=1.0) -> (0:w1350:bool)
                    n603 = case shown="False" w1350 {
                      tunnel: w1348 -> [w1353 w1357]
                      tunnel: w1347 -> [w1352 w1358]
                      tunnel: w1346 -> [w1355 w1361]
                      tunnel: w1345 -> [w1356 w1360]
                      tunnel: [w1354 w1357] -> w1344
                      tunnel: [w1352 w1359] -> w1343
                      tunnel: [w1355 w1361] -> w1342
                      tunnel: [w1356 w1360] -> w1341
                      frame False {
                        n604 = Increment(x=w1353) -> (x+1=w1354:i32)
                      }
                      frame True {
                        n605 = Increment(x=w1358) -> (x+1=w1359:i32)
                      }
                    }
                  }
                  frame True {
                    n606 = Greater?(x=w1371, y=3.0) -> (0:w1370:bool)
                    n607 = case shown="False" w1370 {
                      tunnel: w1369 -> [w1376 w1382]
                      tunnel: w1368 -> [w1375 w1381]
                      tunnel: w1367 -> [w1374 w1378]
                      tunnel: w1366 -> [w1373 w1379]
                      tunnel: [w1376 w1382] -> w1362
                      tunnel: [w1375 w1381] -> w1363
                      tunnel: [w1377 w1378] -> w1365
                      tunnel: [w1373 w1380] -> w1364
                      frame False {
                        n608 = Increment(x=w1374) -> (x+1=w1377:i32)
                      }
                      frame True {
                        n609 = Increment(x=w1379) -> (x+1=w1380:i32)
                      }
                    }
                  }
                }
              }
            }
            n610 = call-poly <vilib>:"DAQmx Create Virtual Channel.vi"("lines"=tag "Dev1/port0/line0") -> ("task out"=w1322:refnum<k21>)  [unwired: 13 in, 1 out]
            n611 = call <vilib>:"DAQmx Start Task.vi"("task/channels in"=w1322) -> ("task out"=w1321:refnum<k21>)  [unwired: 13 in, 1 out]
            n612 = call-poly <vilib>:"DAQmx Write.vi"("task/channels in"=w1321, "data"=TRUE) -> ("task out"=w1320:refnum<k21>)  [unwired: 11 in, 2 out]
            n613 = call <vilib>:"DAQmx Stop Task.vi"("task/channels in"=w1320) -> ()  [unwired: 13 in, 2 out]
          }
        }
        n614 = Increment(x=w306) -> (x+1=w296:i32)
        "Trial" <- w296
        n615 = Divide(x=w296, y=w297) -> (x/y=→"Slide":dbl)
        "Cond. 1" <- w264
        "Cond. 2" <- w262
        "Cond. 3" <- w260
        "Cond. 4" <- w258
      }
    }
    frame #3 {
      n616 = Close File(refnum=w1389) -> ()  [unwired: 1 in, 2 out]
      n617 = Close File(refnum=w1388) -> ()  [unwired: 1 in, 2 out]
      n618 = Close File(refnum=w1391) -> ()  [unwired: 1 in, 2 out]
      n619 = Close File(refnum=w1390) -> ()  [unwired: 1 in, 2 out]
      n620 = call-poly <vilib>:"DAQmx Create Virtual Channel.vi"("physical channels"=tag "Dev1/ao1") -> ("task out"=w1385:refnum<k21>)  [unwired: 13 in, 1 out]
      n621 = call <vilib>:"DAQmx Start Task.vi"("task/channels in"=w1385) -> ("task out"=w1387:refnum<k21>)  [unwired: 13 in, 1 out]
      n622 = call-poly <vilib>:"DAQmx Write.vi"("task/channels in"=w1387, "data"=5.0) -> ("task out"=w1386:refnum<k21>)  [unwired: 11 in, 2 out]
      n623 = call <vilib>:"DAQmx Stop Task.vi"("task/channels in"=w1386) -> ()  [unwired: 13 in, 2 out]
    }
  }
